vi "Turbulence_3.0.vi"() -> ()   [LabVIEW 2018]
uses:
  Quantum Composers 9000 Series.lvlib
  LightField Automation.lvclass
  Mercury iXX.lvlib
  Temperature (Read).vi
  Temperature.lvlib
  Open Temperature Device.vi
  Comms Transport Layer.ctl
  Keithley 2600 Series.lvlib
  Channel.ctl
  DAQmx Read (Counter DBL 1Chan 1Samp).vi
  Catalogue (Read).vi
  System.lvlib
  Open System.vi
panel:
  in  "File Exists":bool
  out "Log":refnum<file>
  in  "Motor free":bool
  in  "RESTART":bool
  out "time string":string
  out "Timestamp":string
  out "Log Error":errorcluster
  in  "CLOSE":bool
  in  "RECORD":bool
  in  "Turbulence":T1(tab)
  in  "New Background":bool
  out "Rate (Hz)":dbl
  out "Incident":dbl
  in  "BIN":u16(ring)=2 items=["1x1", "2x2", "4x4"]
  in  "MODE":u16(ring) items=["Normal", "DIF"]
  in  "Enable":bool
  out "Rate (Hz)":dbl
  out "Detected":dbl
  in  "Script\nEnd":u32=1 step=1
  in  "Sample Space Pump":bool
  in  "Siphon Pump":bool
  in  "Neutron Shutter":bool
  in  "Manual Script Entry (0)":string
  in  "READY":bool
  out "Power (mW)":dbl format="%_3f"
  out "Tank Pressure 2 (Torr)":string="0.0"
  in  "LIGHTFIELD":bool
  in  "SCRIPTING":bool
  in  "Top Coil":bool
  in  "# Frames":i32=1000 min=0 step=1
  in  "On CCD Acc.":i32=3 min=0 step=1
  out "Tank Pressure 1 (Torr)":string="0.0"
  out "Cell Temp (K)":dbl format="%.3f"
  in  "Data folder":path=path "C:/Data"
  out "Cryostat Temp (K)":dbl format="%.3f"
  in  "Data Interval (s)":dbl=0.5 min=0.4 max=10.0 step=0.05
  in  "RUN/STOP":bool
  in  "Bottom Coil":bool
  in  "Bottom Coil (mA)":dbl min=-1000.0 max=1000.0 step=1e-05
  in  "Top Coil (mA)":dbl min=-1000.0 max=1000.0 step=1e-05
  in  "Percent Open":i32 min=0 max=100 step=5
  in  "COOLDOWN":bool
  in  "Script\n#":i32 step=1
  in  "Kill Switch":bool
  in  "DATA":bool
  out "Scripting \nError":T2
  in  "Shutter Mode":u16(ring)=1 items=["Manual"=1, "XGate"=5]
  in  "Time (s)":i32=120 min=1 max=300 step=1
  out "Actual 3He\nTank Pressure":dbl min=0.0 max=100.0 step=5.0 format="%#.1g"
  out "Desired V2\nPressure (3He)":dbl min=0.0 max=100.0 step=5.0 format="%#.1f"
  in  "Desired Tank\nPressure (3He)":dbl min=0.0 max=100.0 step=0.01 format="%#.2f"
  in  "Log Pressure":bool
  out "4He Pressure (Torr)":string="-0.1"
  out "3He Pressure (Torr)":string="1"
  out "Temperature Error":errorcluster={"status"=TRUE, "code"=-1073807339, "source"="VISA Read in Mercury iXX.lvlib:Query (Dynamic).vit->Mercury iXX.lvlib:Query (Low Level).vi:10049->Mercury iXX.lvlib:Query.vi:3960048->Mercury iXX.lvlib:Read (Str).vi:5300004->Mercury iXX.lvlib:System.lvlib:Catalogue (Read).vi->Turbulence.vi"}
  out "File I/O Error":errorcluster
  out "4He Gauge Error":errorcluster={"status"=TRUE, "code"=-1073807343, "source"="VISA Open in Turbulence.vi"}
  out "Heater Error":errorcluster={"status"=FALSE, "code"=1073676293, "source"="VISA Read in Keithley 2600 Series.lvlib:Print Number.vi->Keithley 2600 Series.lvlib:Measure.vi->Turbulence.vi"}
  out "Pulse Generator Error":errorcluster
  out "3He Gauge Error":errorcluster={"status"=FALSE, "code"=1073676293, "source"="VISA Read in 3HeClose.vi->Turbulence.vi"}
  out "Relay Errror":errorcluster
  out "Zaber Motor Error":errorcluster
  out "LightField Error":errorcluster
  out "Shutter Error":errorcluster
  # "Camera Controls"
  # "Temperature Readout"
  # "Pressure Readout"
  # "Neutron Counts"
  # "Automation"
  # "Heater Controls"
  # "Relay Controls"
  # "Needle Valve Control"
  # "Neutron Shutter"
  # "Optical Shutter"
  # "Siphon Pump"
  # "Laser Power Meter"
  # "Sample Space\nPump"
  # "V1 = 4075 mL"
  # "V2 = 15.5 mL"
  # "V3 = 78.8 mL"
  # "Quartz\nCell"
  # "4"
  # "3psi relief"
  # "V1"
  # "4L Tank"
  # "Turbo Pump"
  # "V2"
  # "V3"
  # "3"
  # "10psi relief"
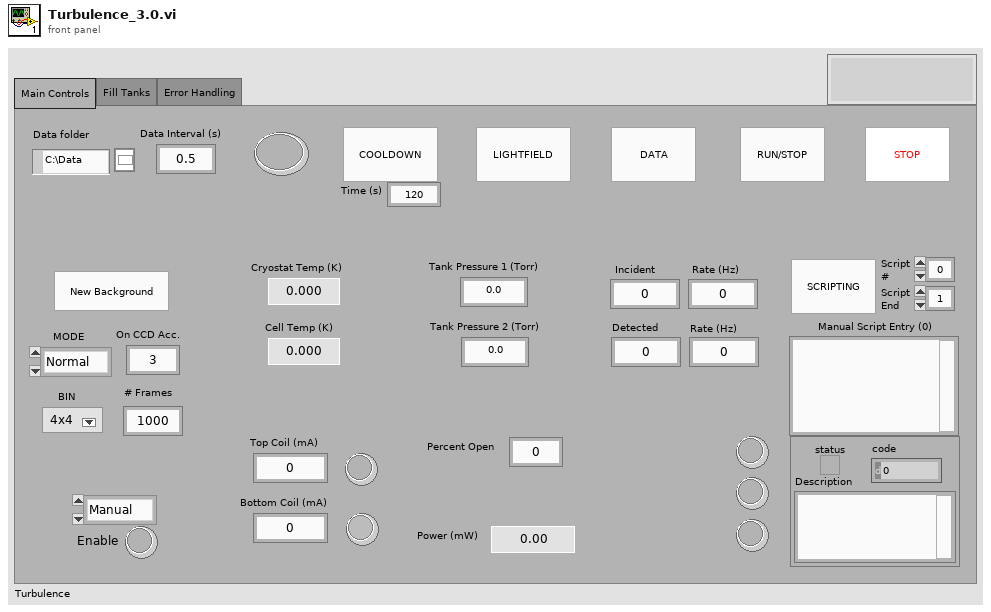
[diagram p1: front panel]
types:
  T1 = enum32{"Main Controls", "Fill Tanks", "Error Handling"}
  T2 = cluster{"status":bool, "code":i32, "Description":string}
  T3 = typedef "Mercury iXX.lvlib/Comms Transport Layer.ctl" = enum16{"Ethernet TCP/IP", "USB", "ISOBus - RS-232", "GPIB"}
  T4 = typedef "Mercury iXX.lvlib/Mercury Reference.ctl" = cluster{"Comms":refnum<visa-resource-name>, "Device ID":string[], "Comms Layer":T3, "Command":string, "Query reference":T5}
  T5 = typedef "Mercury iXX.lvlib/Query Dynamic Reference.ctl" = refnum<vi>
  T6 = enum32{"Current", "Voltage", "IV", "Resistance", "Power"}
  T7 = typedef "Keithley 2600 Series.lvlib/Channel.ctl" = enum32{"Channel A", "Channel B"}
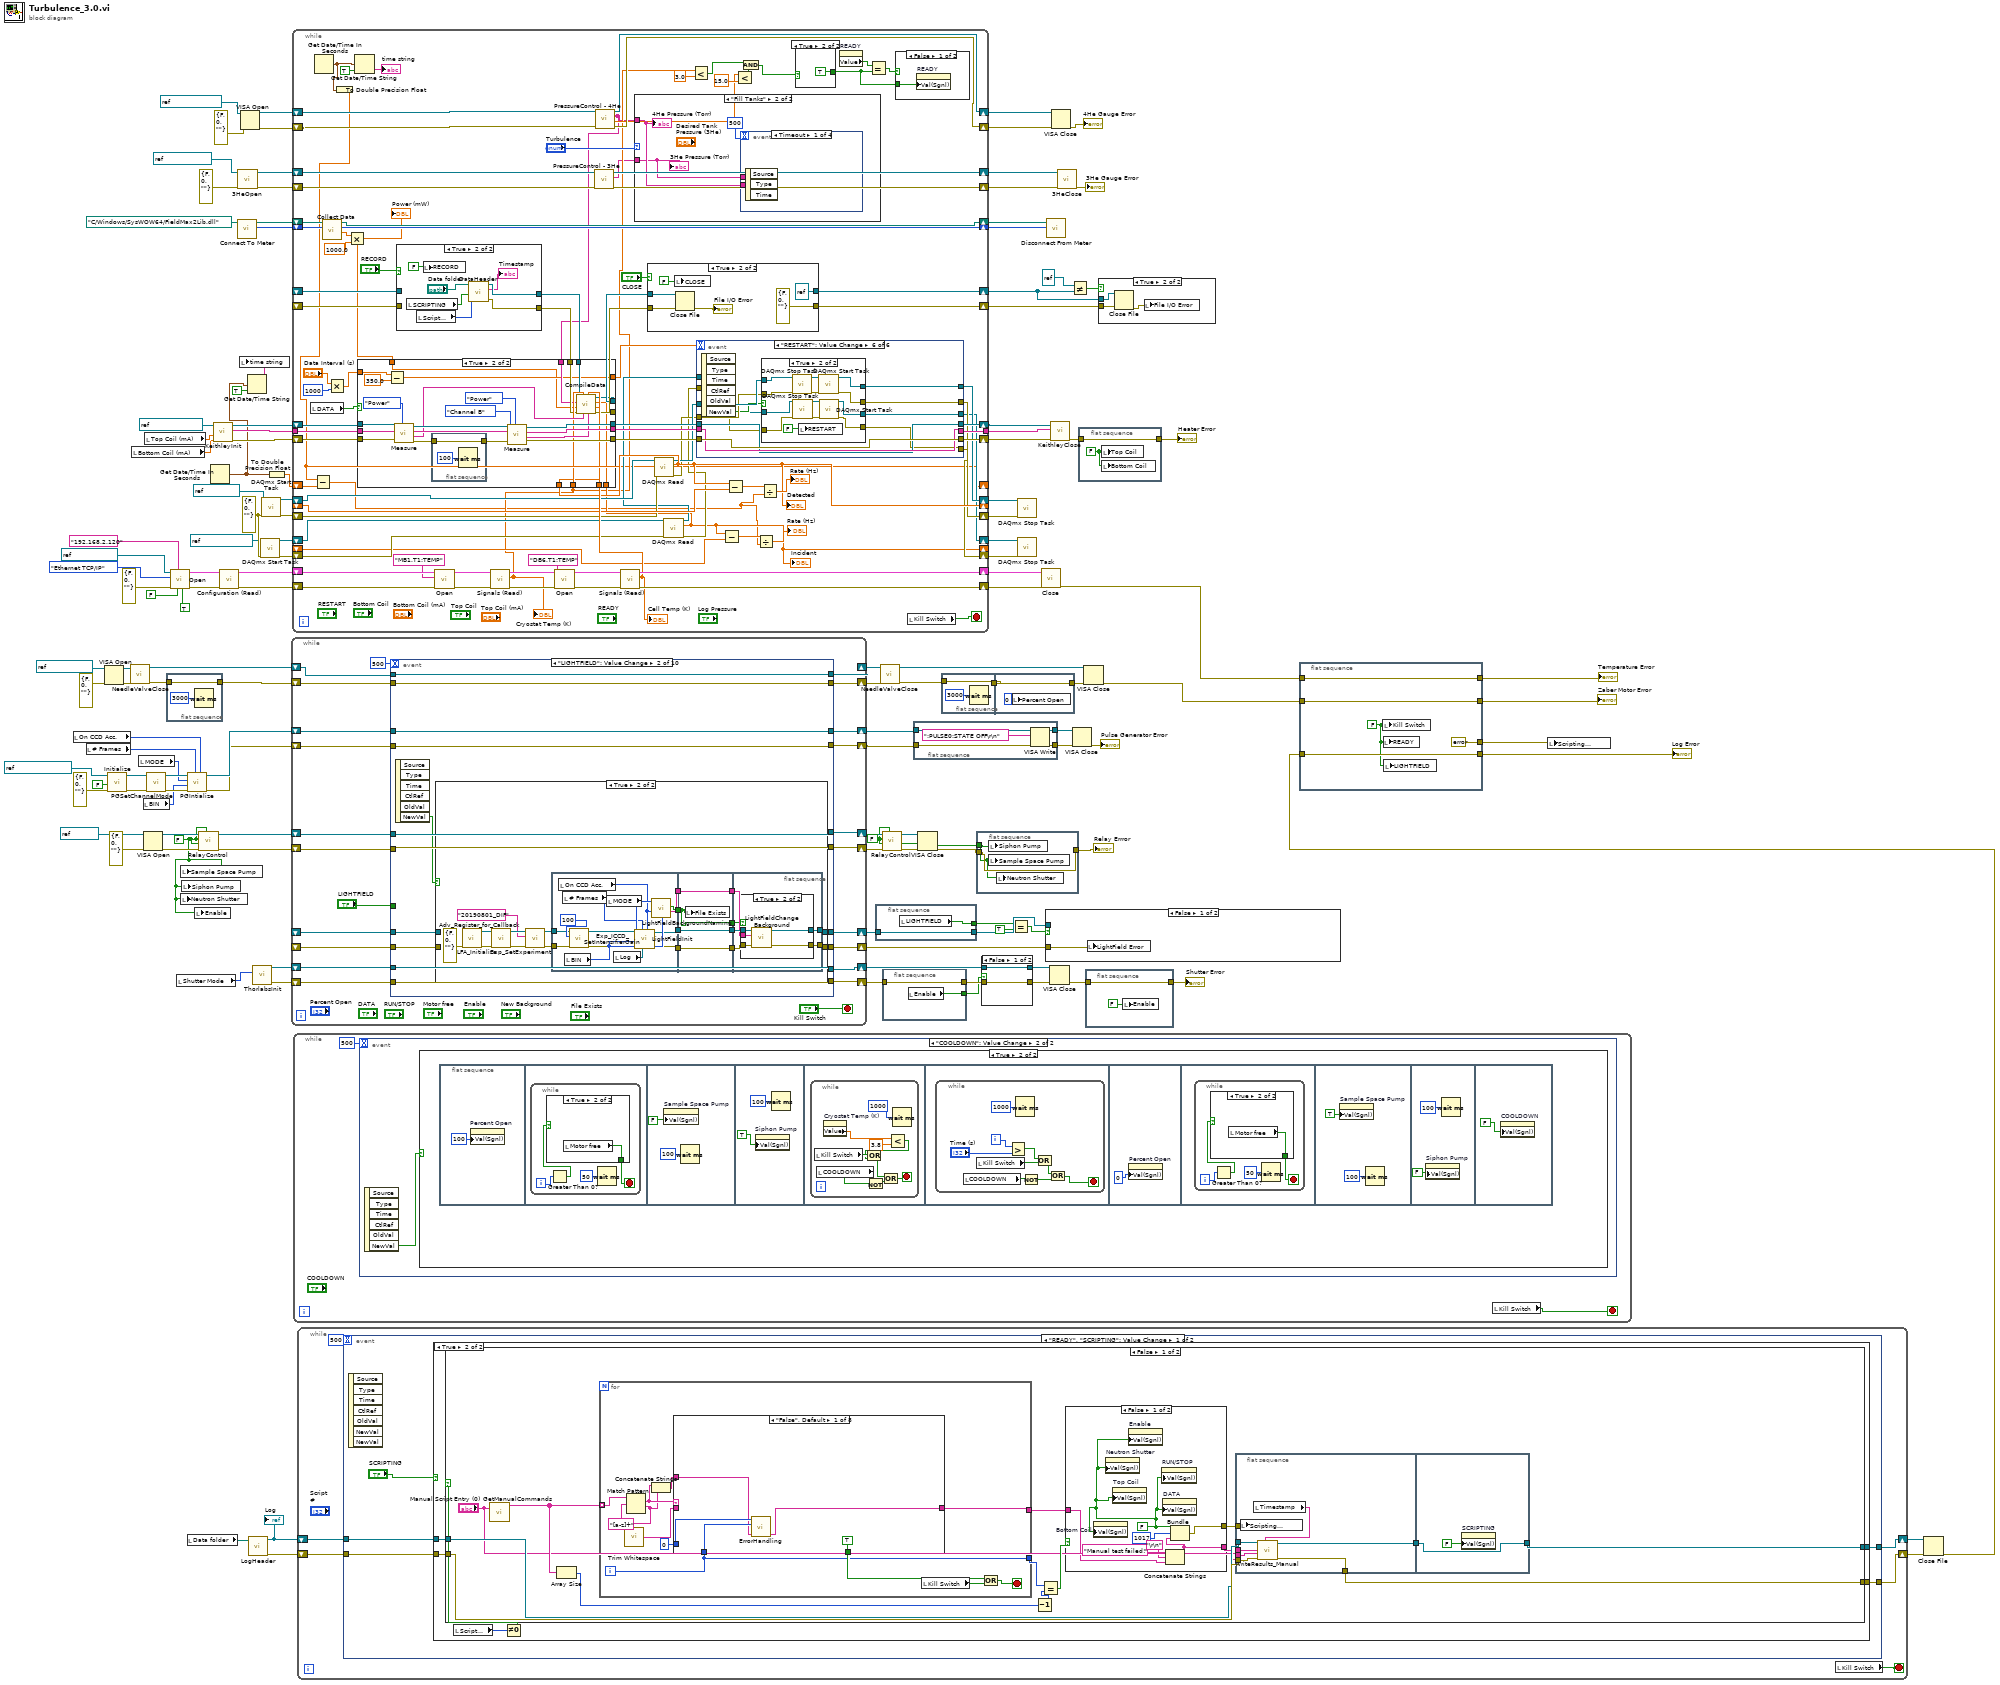
[diagram p0: block diagram]
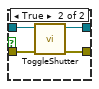
[diagram p2: hidden frame]
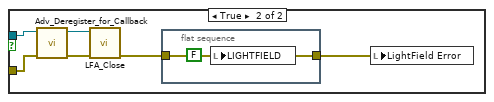
[diagram p3: hidden frame]
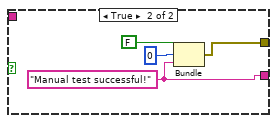
[diagram p5: hidden frame]
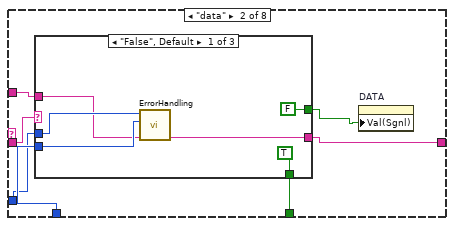
[diagram p6: hidden frame]
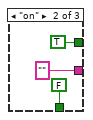
[diagram p7: hidden frame]
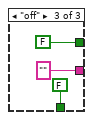
[diagram p8: hidden frame]
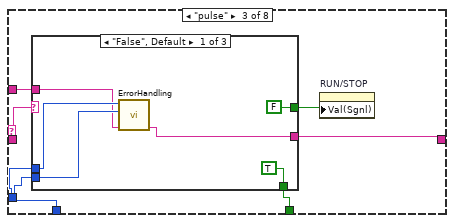
[diagram p9: hidden frame]
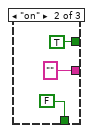
[diagram p10: hidden frame]
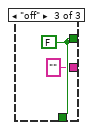
[diagram p11: hidden frame]
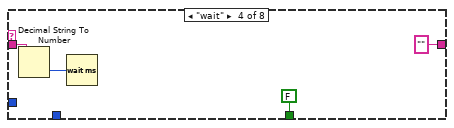
[diagram p12: hidden frame]
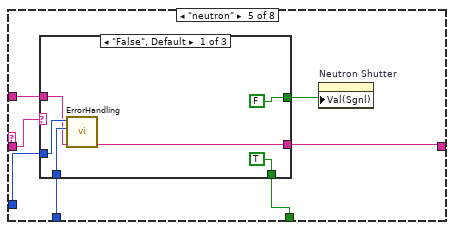
[diagram p13: hidden frame]
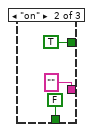
[diagram p14: hidden frame]
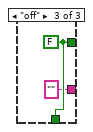
[diagram p15: hidden frame]
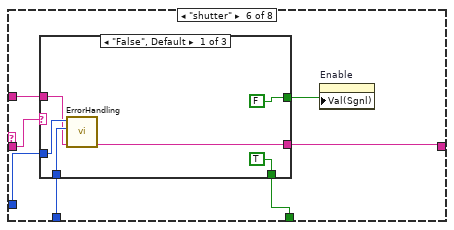
[diagram p16: hidden frame]
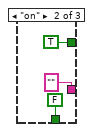
[diagram p17: hidden frame]
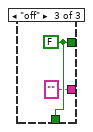
[diagram p18: hidden frame]
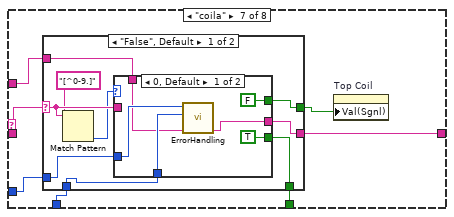
[diagram p19: hidden frame]
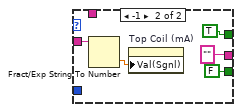
[diagram p20: hidden frame]
diagram:
  w22 = errorcluster {"status"=FALSE, "code"=0, "source"=""} ("error in")
  w60 = FALSE ("Siphon Pump")
  w44 = FALSE ("Siphon Pump")
  n1 = local read "On CCD Acc."() -> (w33:i32)
  n2 = local read "# Frames"() -> (w32:i32)
  n3 = VISA Open(error in (no error)=errorcluster {"status"=FALSE, "code"=0, "source"=""}, VISA resource name=refnum<visa-resource-name> "ZaberMotor") -> (VISA resource name=w39:refnum<visa-resource-name>, error out=w40:errorcluster)  [unwired: 3 in]
  n4 = call "Initialize.vi"("error in (no error)"=errorcluster {"status"=FALSE, "code"=0, "source"=""}, "Reset? (T: Yes)"=FALSE, "VISA resource name"=refnum<visa-resource-name> "PulseGenerator" ("Pulse generater (COM3)")) -> ("error out"=w51:errorcluster, "VISA resource name out"=w49:refnum<visa-resource-name>)  [unwired: 7 in]
  n5 = call "NeedleValveClose.vi"("error in (no error)"=w40, "VISA resource name"=w39) -> ("error out"=w41:errorcluster, "VISA resource name out"=w82:refnum<visa-resource-name>)  [unwired: 8 in]
  n6 = local read "Bottom Coil (mA)"() -> (w94:dbl)
  n7 = local read "MODE"() -> (w30:u16)
  n8 = local read "BIN"() -> (w31:u16)
  n9 = VISA Open(error in (no error)=errorcluster {"status"=FALSE, "code"=0, "source"=""} ("error in (no error) 2"), VISA resource name=refnum<visa-resource-name> "Relays" ("Pressure Gauge")) -> (VISA resource name=w107:refnum<visa-resource-name>, error out=w109:errorcluster)  [unwired: 3 in]
  n10 = local read "Top Coil (mA)"() -> (w95:dbl)
  n11 = call "PGSetChannelMode.vi"("error in"=w51, "VISA resource name"=w49) -> ("error out"=w50:errorcluster, "VISA resource name out"=w48:refnum<visa-resource-name>)  [unwired: 8 in]
  n12 = flat-sequence {
    tunnel: w41 -> [w136]
    tunnel: [w136] -> w83
    frame #0 {
      n13 = Wait (ms)(milliseconds to wait=u32 3000) -> ()  [unwired: 1 out]
    }
  }
  n14 = call-poly "Open.vi"("Clear Previous Connections (False)"=TRUE, "ID Query (True)"=FALSE, "IP Address"="192.168.2.120", "error in (no error)"=errorcluster {"status"=FALSE, "code"=0, "source"=""}, "Comms Layer"=Comms_Transport_Layer."Ethernet TCP/IP", "VISA resource name"=refnum<visa-resource-name> "MercuryiTC") -> ("error out"=w128:errorcluster, "Mercury Reference Out"=w129:T4)  [unwired: 1 in, 3 out]
  n15 = local read "Shutter Mode"() -> (w34:u16)
  n16 = local write "Sample Space Pump"(w44) -> ()
  n17 = local write "Neutron Shutter"(w44) -> ()
  n18 = local write "Siphon Pump"(w44) -> ()
  n19 = local read "Data folder"() -> (w58:path)
  n20 = call "PGIntialize.vi"("On CCD Accumulations"=w33, "Number of Frames"=w32, "error in"=w50, "BIN"=w31, "MODE"=w30, "VISA resource name"=w48) -> ("error out"=w133:errorcluster, "VISA resource name out"=w134:refnum<visa-resource-name>)  [unwired: 4 in]
  n21 = local write "Enable"(w44) -> ()
  n22 = call "RelayControl.vi"("Neutron Shutter"=w44, "Error In"=w109, "Sample Space Pump"=w44, "Siphon Pump"=w44, "Relay In"=w107) -> ("Error Out"=w108:errorcluster, "Relay Out"=w106:refnum<visa-resource-name>)  [unwired: 5 in]
  n23 = Get Date/Time In Seconds() -> (seconds since 1Jan1904=w1:timestamp)
  n24 = call "KeithleyInit.vi"("Bottom Coil (mA)"=w94, "Top Coil (mA)"=w95, "KeithleyVISA In"=refnum<visa-resource-name> "Keithley2614B" ("VISA resource name")) -> ("error out"=w98:errorcluster, "Node Out"=w99:string, "KeithleyVISA Out"=w97:refnum<visa-resource-name>)  [unwired: 6 in]
  n25 = call-poly "Configuration (Read).vi"("error in"=w128, "Mercury Reference In"=w129) -> ("error out"=w124:errorcluster, "Mercury Reference Out"=w125:T4)  [unwired: 6 in, 2 out]
  n26 = call "Connect To Meter.vi"("Location of FieldMax2Lib.dll in"=path "C:/Windows/SysWOW64/FieldMax2Lib.dll") -> ("Meter ID out"=w68:i32, "Location of FieldMax2Lib.dll out"=w67:path)  [unwired: 6 in, 1 out]
  n27 = call "3HeOpen.vi"("error in (no error)"=errorcluster {"status"=FALSE, "code"=0, "source"=""} ("error in (no error) 2"), "VISA resource name"=refnum<visa-resource-name> "3HePressure" ("Pressure Gauge")) -> ("error out"=w111:errorcluster, "VISA resource name out"=w110:refnum<visa-resource-name>)  [unwired: 8 in]
  n28 = VISA Open(error in (no error)=errorcluster {"status"=FALSE, "code"=0, "source"=""} ("error in (no error) 2"), VISA resource name=refnum<visa-resource-name> "TankPressure" ("Pressure Gauge")) -> (VISA resource name=w121:refnum<visa-resource-name>, error out=w122:errorcluster)  [unwired: 3 in]
  n29 = Get Date/Time String(seconds (now)=w1, want seconds? (F)=TRUE) -> (time string=w2:string)  [unwired: 1 in, 1 out]
  n30 = local write "time string"(w2) -> ()
  n31 = call "LogHeader.vi"("Data folder"=w58) -> ("error out"=w56:errorcluster, "refnum out"=w57:refnum<file>)  [unwired: 9 in]
  "Log" <- w57
  n32 = call "ThorlabsInit.vi"("Shutter Mode"=w34) -> ("error out"=w45:errorcluster, "VISA resource name out"=w46:refnum<visa-resource-name>)  [unwired: 9 in]
  n33 = call "DAQmx Start Task.vi"("task/channels in"=refnum<k21> "IncidentBeam", "error in"=w22) -> ("task out"=w24:refnum<k21>, "error out"=w23:errorcluster)  [unwired: 12 in]
  n34 = call "DAQmx Start Task.vi"("task/channels in"=refnum<k21> "Detector", "error in"=w22) -> ("task out"=w27:refnum<k21>, "error out"=w26:errorcluster)  [unwired: 12 in]
  n35 = To Double Precision Float(number=w1) -> (double precision float=w4:dbl)
  n36 = while {
    shift-right: [w159] -> w11
    shift-left: _ -> [w157]
    shift-right: [w160] -> w18
    shift-left: _ -> [w158]
    shift-right: [w153] -> w76
    shift-left: w134 -> [w155]
    shift-right: [w154] -> w77
    shift-left: w133 -> [w156]
    shift-right: [w149] -> w81
    shift-left: w108 -> [w152]
    shift-right: [w150] -> w79
    shift-left: w106 -> [w151]
    shift-right: [w144] -> w112
    shift-left: w83 -> [w147]
    shift-right: [w145] -> w113
    shift-left: w82 -> [w146]
    shift-right: [w141] -> w14
    shift-left: w46 -> [w138]
    shift-right: [w140] -> w7
    shift-left: w45 -> [w139]
    stop <- "Kill Switch" stop-if-true
    n37 = event shown="[1] \"LIGHTFIELD\": Value Change" {
      selector: _ -> [_ _ _ _ _ _ _ _ _ _]
      dyn-events: _ -> [_ _ _ _ _ _ _ _ _ _]
      timeout: 500 -> [_ _ _ _ _ _ _ _ _ _]
      tunnel: w156 -> [w168 w177 w253 w296 w314 w361 w424 w443 w458 w481]
      tunnel: w155 -> [w167 w176 w254 w297 w313 w362 w425 w442 w457 w480]
      tunnel: w158 -> [w169 w180 w244 w288 w316 w365 w422 w446 w462 w472]
      tunnel: w157 -> [w170 w181 w245 w289 w317 w366 w423 w447 w461 w473]
      tunnel: [w169 w182 w243 w288 w316 w353 w422 w446 w462 w472] -> w160
      tunnel: [w170 w183 w242 w289 w317 w345 w423 w447 w461 w473] -> w159
      tunnel: [w168 w177 w256 w296 w314 w351 w424 w443 w458 w478] -> w154
      tunnel: [w167 w176 w255 w297 w313 w358 w425 w442 w457 w479] -> w153
      tunnel: w152 -> [w165 w178 w250 w294 w319 w360 w431 w445 w460 w474]
      tunnel: w151 -> [w166 w179 w251 w295 w318 w359 w430 w444 w459 w475]
      tunnel: [w166 w179 w251 w295 w318 w359 w427 w444 w459 w475] -> w150
      tunnel: [w165 w178 w250 w294 w319 w360 w426 w445 w460 w474] -> w149
      tunnel: w147 -> [w164 w175 w249 w298 w302 w364 w421 w441 w456 w476]
      tunnel: w146 -> [w163 w174 w248 w299 w315 w363 w420 w440 w455 w477]
      tunnel: [w163 w174 w248 w299 w312 w363 w420 w440 w455 w477] -> w145
      tunnel: [w164 w175 w249 w298 w304 w364 w421 w441 w456 w476] -> w144
      tunnel: "LIGHTFIELD" -> [_ _ w241 w293 _ w347 _ _ _ w468]
      tunnel: w138 -> [w161 w172 w247 w291 w310 w357 w418 w439 w466 w471]
      tunnel: w139 -> [w162 w171 w246 w290 w309 w356 w417 w438 w465 w470]
      tunnel: [w161 w172 w247 w291 w310 w357 w418 w436 w463 w471] -> w141
      tunnel: [w162 w171 w246 w290 w309 w356 w417 w437 w464 w470] -> w140
      event Timeout {
        n38 = event-data() -> ()  [unwired: 1 in, 3 out]
      }
      event "LIGHTFIELD": Value Change {
        n39 = event-data() -> ("NewVal"=w173:bool)  [unwired: 1 in, 5 out]
        n40 = case shown="True" w173 {
          tunnel: [refnum<class "LightField Automation.lvclass"> refnum ("LightField Automation out") w199] -> w183
          tunnel: [errorcluster {"status"=FALSE, "code"=0, "source"=""} ("error out") w198] -> w182
          tunnel: w181 -> [w187 _]
          tunnel: w180 -> [w186 _]
          frame False {
            n41 = call "Adv_Deregister_for_Callback.vi"("error in (no error)"=w186, "LightField Automation in"=w187) -> ("error out"=w189:errorcluster, "LightField Automation out"=w190:refnum<class "LightField Automation.lvclass">)  [unwired: 8 in]
            n42 = call "LFA_Close.vi"("error in (no error)"=w189, "LightField Automation in"=w190) -> ("error out"=→"LightField Error":errorcluster)  [unwired: 8 in, 1 out]
          }
          frame True {
            n43 = call "LFA_Initialize.vi"("error in (no error)"=errorcluster {"status"=FALSE, "code"=0, "source"=""}) -> ("error out"=w208:errorcluster, "LightField Automation out"=w207:refnum<class "LightField Automation.lvclass">)  [unwired: 9 in]
            n44 = call "Adv_Register_for_Callback.vi"("error in (no error)"=w208, "LightField Automation in"=w207) -> ("error out"=w206:errorcluster, "LightField Automation out"=w205:refnum<class "LightField Automation.lvclass">)  [unwired: 8 in]
            n45 = call "Exp_SetExperiment.vi"("error in (no error)"=w206, "ExperimentName"="20190801_DIF", "LightField Automation in"=w205) -> ("error out"=w192:errorcluster, "LightField Automation out"=w191:refnum<class "LightField Automation.lvclass">)  [unwired: 7 in]
            n46 = flat-sequence {
              tunnel: [w211] -> w196
              tunnel: [w210] -> w195
              tunnel: [w209] -> w194
              tunnel: [w212] -> w193
              tunnel: w192 -> [w215]
              tunnel: w191 -> [w213]
              tunnel: [w226] -> w202
              tunnel: [w225] -> w201
              tunnel: [w224] -> w200
              tunnel: [w223] -> w197
              tunnel: w196 -> [w223]
              tunnel: w195 -> [w226]
              tunnel: w194 -> [w225]
              tunnel: w193 -> [w224]
              tunnel: w202 -> [w231]
              tunnel: w201 -> [w232]
              tunnel: w200 -> [w230]
              tunnel: [w229] -> w199
              tunnel: [w228] -> w198
              tunnel: w197 -> [w227]
              frame #0 {
                n47 = local read "On CCD Acc."() -> (w221:i32)
                n48 = local read "# Frames"() -> (w219:i32)
                n49 = local read "BIN"() -> (w220:u16)
                n50 = call "Exp_ICCD_SetIntensifierGain.vi"("error in (no error)"=w215, "Intensifier Gain"=100, "LightField Automation in"=w213) -> ("error out"=w217:errorcluster, "LightField Automation out"=w216:refnum<class "LightField Automation.lvclass">)  [unwired: 7 in]
                n51 = local read "MODE"() -> (w222:u16)
                n52 = local read "Log"() -> (w218:refnum<file>)
                n53 = call "LightFieldInit.vi"("On CCD Accumulations"=w221, "File Path"=w218, "Number of Frames"=w219, "error in"=w217, "BIN"=w220, "MODE"=w222, "LightField Automation in"=w216) -> ("error out"=w210:errorcluster, "LightField Automation out"=w209:refnum<class "LightField Automation.lvclass">)  [unwired: 3 in]
                n54 = call "LightFieldBackgroundNaming.vi"("On CCD Acc."=w221, "BIN"=w220, "MODE"=w222) -> ("FilePath"=w212:string, "Exists"=w211:bool)  [unwired: 6 in, 1 out]
              }
              frame #1 {
                n55 = local write "File Exists"(w223) -> ()
              }
              frame #2 {
                n56 = case shown="True" w227 {
                  tunnel: w232 -> [w235 w240]
                  tunnel: w231 -> [w234 w239]
                  tunnel: w230 -> [_ w238]
                  tunnel: [w235 w237] -> w229
                  tunnel: [w234 w236] -> w228
                  frame False {
                    n57 = property on="New Background" class="Bool (strict)"("Val(Sgnl)"=TRUE ("Value (Signaling)")) -> ()  [unwired: 2 in, 2 out]
                  }
                  frame True {
                    n58 = call "LightFieldChangeBackground.vi"("error in"=w239, "FilePath"=w238, "LightField Automation in"=w240) -> ("error out"=w236:errorcluster, "LightField Automation out"=w237:refnum<class "LightField Automation.lvclass">)  [unwired: 7 in]
                  }
                }
              }
            }
          }
        }
      }
      event "RUN/STOP": Value Change {
        n59 = event-data() -> ("NewVal"=w252:bool)  [unwired: 1 in, 5 out]
        n60 = case shown="False" w252 {
          tunnel: [w260 w273] -> w256
          tunnel: [w261 w272] -> w255
          tunnel: w254 -> [w262 w271]
          tunnel: w253 -> [w263 w270]
          tunnel: w245 -> [w258 w268]
          tunnel: w244 -> [w257 w267]
          tunnel: [w257 w266] -> w243
          tunnel: [w258 w265] -> w242
          tunnel: w241 -> [_ w264]
          frame False {
            n61 = VISA Write(VISA resource name=w262, write buffer=":PULSE0:STATE OFF\r\n" ("format string"), error in (no error)=w263) -> (VISA resource name out=w261:refnum<visa-resource-name>, error out=w260:errorcluster)  [unwired: 1 out]
          }
          frame True {
            n62 = case shown="True" w264 {
              tunnel: w267 -> [w274 w283]
              tunnel: w268 -> [w275 w281]
              tunnel: [w275 w285] -> w265
              tunnel: [w274 w284] -> w266
              frame False {
              }
              frame True {
                n63 = local read "MODE"() -> (w278:u16)
                n64 = local read "SCRIPTING"() -> (w276:bool)
                n65 = local read "BIN"() -> (w279:u16)
                n66 = case shown="True" w276 {
                  tunnel: [-1 ("Script\n#") w287] -> w277
                  frame False {
                  }
                  frame True {
                    n67 = local read "Script\n#"() -> (w287:i32)
                  }
                }
                n68 = call "LightFieldFileNaming.vi"("Script#"=w277, "error in"=w283, "BIN"=w279, "MODE"=w278, "LightField Automation in"=w281) -> ("error out"=w282:errorcluster, "LightField Automation out"=w280:refnum<class "LightField Automation.lvclass">)  [unwired: 5 in]
                n69 = call "LFA_Acquire.vi"("error in (no error)"=w282, "LightField Automation in"=w280) -> ("error out"=w284:errorcluster, "LightField Automation out"=w285:refnum<class "LightField Automation.lvclass">)  [unwired: 8 in]
              }
            }
            n70 = VISA Write(VISA resource name=w271, write buffer=":PULSE0:STATE ON\r\n" ("format string"), error in (no error)=w270) -> (VISA resource name out=w272:refnum<visa-resource-name>, error out=w273:errorcluster)  [unwired: 1 out]
          }
        }
      }
      event "DATA": Value Change {
        n71 = event-data() -> ("NewVal"=w292:bool)  [unwired: 1 in, 5 out]
        n72 = case shown="True" w292 {
          tunnel: w293 -> [_ _]
          frame False {
            n73 = local write "CLOSE"(TRUE ("CLOSE")) -> ()
          }
          frame True {
            n74 = local write "RECORD"(TRUE ("RECORD")) -> ()
          }
        }
      }
      event "Percent Open": Value Change {
        n75 = event-data() -> ("OldVal"=w311:i32, "NewVal"=w320:i32)  [unwired: 1 in, 4 out]
        n76 = flat-sequence {
          tunnel: w302 -> [w322]
          tunnel: [w322] -> w303
          frame #0 {
            n77 = property on="Motor free" class="Bool (strict)"("Val(Sgnl)"=FALSE ("Value (Signaling)")) -> ()  [unwired: 2 in, 2 out]
          }
        }
        n78 = Subtract(x=w320, y=w311) -> (x-y=w306:i32)
        n79 = Greater Than 0?(x=w306) -> (x > 0?=w307:bool)
        n80 = Equal To 0?(x=w320) -> (x = 0?=w308:bool)
        n81 = case shown="False" w308 {
          tunnel: w315 -> [w328 w344]
          tunnel: w303 -> [w329 w343]
          tunnel: [w327 w342] -> w312
          tunnel: [w326 w341] -> w305
          tunnel: w307 -> [w330 _]
          tunnel: w306 -> [w325 _]
          frame False {
            n82 = case shown="True" w330 {
              tunnel: w329 -> [w334 w340]
              tunnel: w328 -> [w335 w339]
              tunnel: [w333 w338] -> w327
              tunnel: [w332 w337] -> w326
              tunnel: w325 -> [w331 w336]
              frame False {
                n83 = call "NeedleValveClose - Encoder.vi"("error in (no error)"=w334, "Percent Difference"=w331, "VISA resource name"=w335) -> ("error out"=w332:errorcluster, "VISA resource name out"=w333:refnum<visa-resource-name>)  [unwired: 7 in]
              }
              frame True {
                n84 = call "NeedleValveOpen - Encoder.vi"("error in (no error)"=w340, "Percent Difference"=w336, "VISA resource name"=w339) -> ("error out"=w337:errorcluster, "VISA resource name out"=w338:refnum<visa-resource-name>)  [unwired: 7 in]
              }
            }
          }
          frame True {
            n85 = call "NeedleValveClose.vi"("error in (no error)"=w343, "VISA resource name"=w344) -> ("error out"=w341:errorcluster, "VISA resource name out"=w342:refnum<visa-resource-name>)  [unwired: 8 in]
          }
        }
        n86 = flat-sequence {
          tunnel: w305 -> [w324]
          tunnel: [w324] -> w304
          frame #0 {
            n87 = property on="Motor free" class="Bool (strict)"("Val(Sgnl)"=TRUE ("Value (Signaling)")) -> ()  [unwired: 2 in, 2 out]
          }
        }
      }
      event "On CCD Acc.", "# Frames", "MODE", "BIN": Value Change {
        n88 = event-data() -> ()  [unwired: 1 in, 4 out]
        n89 = case shown="True" w347 {
          tunnel: w366 -> [w405 w413]
          tunnel: w365 -> [w406 w414]
          tunnel: [w405 w412] -> w346
          tunnel: [w406 w411] -> w354
          tunnel: "On CCD Acc." -> [_ w409]
          tunnel: "# Frames" -> [_ w410]
          tunnel: "BIN" -> [_ w408]
          tunnel: "MODE" -> [_ w407]
          frame False {
          }
          frame True {
            n90 = call "LightFieldParams.vi"("On CCD Accumulations"=w409, "Number of Frames"=w410, "error in"=w414, "BIN"=w408, "MODE"=w407, "LightField Automation in"=w413) -> ("error out"=w411:errorcluster, "LightField Automation out"=w412:refnum<class "LightField Automation.lvclass">)  [unwired: 4 in]
          }
        }
        n91 = call "PGIntialize.vi"("On CCD Accumulations"="On CCD Acc.", "Number of Frames"="# Frames", "error in"=w361, "BIN"="BIN", "MODE"="MODE", "VISA resource name"=w362) -> ("error out"=w352:errorcluster, "VISA resource name out"=w358:refnum<visa-resource-name>)  [unwired: 4 in]
        n92 = case shown="True" w347 {
          tunnel: w354 -> [w369 w378]
          tunnel: [w369 w377] -> w353
          tunnel: w352 -> [w368 w376]
          tunnel: [w368 w375] -> w351
          tunnel: "On CCD Acc." -> [_ w374]
          tunnel: "BIN" -> [_ w373]
          tunnel: "MODE" -> [_ w372]
          tunnel: w346 -> [w367 w371]
          tunnel: [w367 w370] -> w345
          frame False {
          }
          frame True {
            n93 = flat-sequence {
              tunnel: w378 -> [w381]
              tunnel: [w380] -> w377
              tunnel: w376 -> [w389]
              tunnel: [w389] -> w375
              tunnel: w374 -> [w388]
              tunnel: w373 -> [w387]
              tunnel: w372 -> [w386]
              tunnel: w371 -> [w382]
              tunnel: [w379] -> w370
              frame #0 {
                n94 = call "LightFieldBackgroundNaming.vi"("On CCD Acc."=w388, "BIN"=w387, "MODE"=w386) -> ("FilePath"=w383:string, "Exists"=w385:bool)  [unwired: 6 in, 1 out]
                n95 = flat-sequence {
                  tunnel: w385 -> [w390]
                  tunnel: [w390] -> w384
                  tunnel: w384 -> [w396]
                  tunnel: w383 -> [w395]
                  tunnel: w382 -> [w394]
                  tunnel: w381 -> [w393]
                  tunnel: [w392] -> w380
                  tunnel: [w391] -> w379
                  frame #0 {
                    n96 = local write "File Exists"(w390) -> ()
                  }
                  frame #1 {
                    n97 = case shown="False" w396 {
                      tunnel: w395 -> [_ w404]
                      tunnel: w394 -> [w398 w403]
                      tunnel: w393 -> [w397 w402]
                      tunnel: [w397 w401] -> w392
                      tunnel: [w398 w400] -> w391
                      frame False {
                        n98 = property on="New Background" class="Bool (strict)"("Val(Sgnl)"=TRUE ("Value (Signaling)")) -> ()  [unwired: 2 in, 2 out]
                      }
                      frame True {
                        n99 = call "LightFieldChangeBackground.vi"("error in"=w402, "FilePath"=w404, "LightField Automation in"=w403) -> ("error out"=w401:errorcluster, "LightField Automation out"=w400:refnum<class "LightField Automation.lvclass">)  [unwired: 7 in]
                      }
                    }
                  }
                }
              }
            }
          }
        }
      }
      event "Siphon Pump", "Sample Space Pump", "Neutron Shutter": Value Change {
        n100 = event-data() -> ("CtlRef"=w416:refnum<vi>)  [unwired: 1 in, 5 out]
        n101 = property class="Bool (strict)"(reference=w416) -> ("Label.Text"=w415:string)  [unwired: 1 in, 2 out]
        n102 = call "RelayControl.vi"("Neutron Shutter"="Neutron Shutter", "Error In"=w431, "Sample Space Pump"="Sample Space Pump", "Siphon Pump"="Siphon Pump", "Relay In"=w430) -> ("Error Out"=w426:errorcluster, "Relay Out"=w427:refnum<visa-resource-name>)  [unwired: 5 in]
        n103 = case shown="\"Neutron Shutter\"" w415 {
          frame "0", Default {
          }
          frame "Neutron Shutter" {
            n104 = property on="RESTART" class="Bool (strict)"("Val(Sgnl)"=TRUE ("RESTART")) -> ()  [unwired: 2 in, 2 out]
          }
        }
      }
      event "Enable": Value Change {
        n105 = event-data() -> ("OldVal"=w434:bool, "NewVal"=w435:bool)  [unwired: 1 in, 4 out]
        n106 = Not Equal?(x=w434, y=w435) -> (x != y?=w433:bool)
        n107 = case shown="True" w433 {
          tunnel: w439 -> [w449 w453]
          tunnel: w438 -> [w448 w452]
          tunnel: [w448 w451] -> w437
          tunnel: [w449 w450] -> w436
          frame False {
          }
          frame True {
            n108 = call "ToggleShutter.vi"("error in"=w452, "VISA resource name"=w453) -> ("error out"=w451:errorcluster, "VISA resource name out"=w450:refnum<visa-resource-name>)  [unwired: 8 in]
          }
        }
      }
      event "Shutter Mode": Value Change {
        n109 = event-data() -> ()  [unwired: 1 in, 6 out]
        n110 = call "ThorlabsMode.vi"("error in"=w465, "Mode"="Shutter Mode", "VISA resource name"=w466) -> ("error out"=w464:errorcluster, "VISA resource name out"=w463:refnum<visa-resource-name>)  [unwired: 7 in]
      }
      event "New Background": Value Change {
        n111 = event-data() -> ("NewVal"=w469:bool)  [unwired: 1 in]
        n112 = And(x=w469, y=w468) -> (x .and. y?=w467:bool)
        n113 = case shown="True" w467 {
          tunnel: w481 -> [w482 w493]
          tunnel: w480 -> [w483 w494]
          tunnel: [w483 w491] -> w479
          tunnel: [w482 w485] -> w478
          frame False {
          }
          frame True {
            n114 = local read "On CCD Acc."() -> (w492:i32)
            n115 = local read "MODE"() -> (w488:u16)
            n116 = local read "File Exists"() -> (w484:bool)
            n117 = local read "BIN"() -> (w487:u16)
            n118 = call "LightFieldAcquireBackground.vi"("File Exists"=w484, "On CCD Acc."=w492, "error in"=w493, "BIN"=w487, "MODE"=w488, "VISA resource name"=w494) -> ("error out"=w490:errorcluster, "VISA resource name out"=w489:refnum<visa-resource-name>)  [unwired: 4 in]
            n119 = call "PGResetCameraWait.vi"("error in"=w490, "BIN"=w487, "MODE"=w488, "VISA resource name"=w489) -> ("error out"=w486:errorcluster, "VISA resource name out"=w491:refnum<visa-resource-name>)  [unwired: 6 in]
            n120 = flat-sequence {
              tunnel: w486 -> [w496]
              tunnel: [w496] -> w485
              frame #0 {
                n121 = local write "New Background"(FALSE ("New Background")) -> ()
                n122 = local write "File Exists"(TRUE ("File Exists")) -> ()
              }
            }
          }
        }
      }
    }
  }
  n123 = while {
    shift-right: [w588] -> w126
    shift-left: w125 -> [w587]
    shift-right: [w589] -> w127
    shift-left: w124 -> [w586]
    shift-right: [w583] -> w117
    shift-left: w122 -> [w585]
    shift-right: [w582] -> w116
    shift-left: w121 -> [w584]
    shift-right: [w581] -> w62
    shift-left: _ -> [w579]
    shift-right: [w580] -> w61
    shift-left: _ -> [w578]
    shift-right: [w575] -> w86
    shift-left: w97 -> [w577]
    shift-right: [w574] -> w88
    shift-left: w98 -> [w573]
    shift-right: [w571] -> w101
    shift-left: w111 -> [w572]
    shift-right: [w569] -> w102
    shift-left: w110 -> [w570]
    tunnel: w99 -> [w576]
    tunnel: [w545] -> w87
    shift-right: [w542] -> w66
    shift-left: w68 -> [w544]
    shift-right: [w541] -> w65
    shift-left: w67 -> [w543]
    shift-right: [w530] -> _
    shift-left: _ -> [w534]
    shift-right: [w529] -> w28
    shift-left: w26 -> [w526]
    shift-right: [w528] -> w29
    shift-left: w27 -> [w527]
    shift-right: [w520] -> w20
    shift-left: w24 -> [w523]
    shift-right: [w521] -> w19
    shift-left: w23 -> [w522]
    shift-right: [w514] -> _
    shift-left: _ -> [w516]
    shift-right: [w498] -> _
    shift-left: w4 -> [w500]
    stop <- w535 stop-if-true
    n124 = local read "DATA"() -> (w540:bool)
    n125 = Get Date/Time In Seconds() -> (seconds since 1Jan1904=w502:timestamp)
    n126 = call "Collect Data.vi"("Location of FieldMax2Lib.dll in"=w543, "Meter ID in"=w544) -> ("Location of FieldMax2Lib.dll out"=w541:path, "Meter ID out"=w542:i32, "Measurement"=w538:sgl)  [unwired: 5 in, 1 out]
    n127 = Multiply(x="Data Interval (s)", y=u32 1000 ("millisecond multiple")) -> (x*y=w546:dbl)
    n128 = To Double Precision Float(number=w502) -> (double precision float=w498:dbl)
    n129 = Subtract(x=w498, y=w500) -> (x-y=w499:dbl)
    n130 = Multiply(x=w538, y=1000.0) -> (x*y=w537:dbl)
    "Power (mW)" <- w537
    n131 = Get Date/Time String(seconds (now)=w502, want seconds? (F)=TRUE) -> (time string=→"time string":string)  [unwired: 1 in, 1 out]
    n132 = case shown="True" "RECORD" {
      tunnel: w579 -> [w637 _]
      tunnel: w578 -> [w638 _]
      tunnel: [w638 w643] -> w549
      tunnel: [w637 w642] -> w550
      frame False {
      }
      frame True {
        n133 = local read "SCRIPTING"() -> (w641:bool)
        n134 = local read "Script\n#"() -> (w640:i32)
        n135 = local write "RECORD"(FALSE ("RECORD")) -> ()
        n136 = call "DataHeader.vi"("Script #"=w640, "Scripting"=w641, 11:"Data folder") -> ("error out"=w642:errorcluster, "Timestamp"=→"Timestamp":string, "refnum out"=w643:refnum<file>)  [unwired: 6 in]
      }
    }
    n137 = call-poly "Open.vi"("error in (no error)"=w586, "Device Identifier"="MB1.T1:TEMP", "Mercury Reference In"=w587) -> ("error out"=w562:errorcluster, "Mercury Reference Out"=w561:T4)  [unwired: 7 in]
    n138 = call-poly "Signals (Read).vi"("error in"=w562, "Mercury Reference In"=w561) -> ("error out"=w559:errorcluster, "Temperature"=w510:dbl, "Mercury Reference Out"=w560:T4)  [unwired: 5 in, 2 out]
    "Cryostat Temp (K)" <- w510
    n139 = call-poly "Open.vi"("error in (no error)"=w559, "Device Identifier"="DB6.T1:TEMP", "Mercury Reference In"=w560) -> ("error out"=w557:errorcluster, "Mercury Reference Out"=w558:T4)  [unwired: 7 in]
    n140 = call "PressureControl - 3He.vi"("error in (no error)"=w572, "VISA resource name"=w570) -> ("error out"=w571:errorcluster, "3HePressure (Torr)"=w504:string, "VISA resource name out"=w569:refnum<visa-resource-name>)  [unwired: 7 in]
    n141 = call "PressureControl - 4He.vi"("error in (no error)"=w585, "VISA resource name"=w584) -> ("error out"=w583:errorcluster, "Pressure"=w552:dbl, "Pressure (Torr)"=w505:string, "VISA resource name out"=w582:refnum<visa-resource-name>)  [unwired: 6 in]
    n142 = call-poly "Signals (Read).vi"("error in"=w557, "Mercury Reference In"=w558) -> ("error out"=w589:errorcluster, "Temperature"=w551:dbl, "Mercury Reference Out"=w588:T4)  [unwired: 5 in, 2 out]
    "Cell Temp (K)" <- w551
    n143 = case shown="\"Fill Tanks\"" "Turbulence" {
      tunnel: w505 -> [w646 w649]
      tunnel: w504 -> [w647 w648]
      frame "Main Controls", Default {
        "Tank Pressure 2 (Torr)" <- w647
        "Tank Pressure 1 (Torr)" <- w646
      }
      frame "Fill Tanks" {
        n144 = event shown="[0] Timeout" {
          selector: _ -> [_ _ _ _]
          dyn-events: _ -> [_ _ _ _]
          timeout: 500 ("Numeric") -> [_ _ _ _]
          tunnel: w648 -> [_ _ _ w655]
          tunnel: w649 -> [_ _ _ w657]
          event Timeout {
            n145 = event-data() -> ()  [unwired: 1 in, 3 out]
          }
          event "Desired Tank\nPressure (3He)": Value Change {
            n146 = event-data() -> ("NewVal"=w651:dbl)  [unwired: 1 in]
            n147 = call "3HePressureCalculator.vi"("Desired Tank\nPressure (3He)"=w651) -> ("V2 Pressure (3He)"=→"Desired V2\nPressure (3He)":dbl)  [unwired: 10 in]
          }
          event "3He Pressure (Torr)": Value Change {
            n148 = event-data() -> ("NewVal"=w653:string)  [unwired: 1 in]
            n149 = call "3HeActualPressure.vi"("3He Pressure (Torr)"=w653) -> ("Actual 3He\nTank Pressure"=→"Actual 3He\nTank Pressure":dbl)  [unwired: 10 in]
          }
          event "Log Pressure": Value Change {
            n150 = event-data() -> ("NewVal"=w656:bool)  [unwired: 1 in, 1 out]
            n151 = call "SaveTankData.vi"("Log Pressure"=w656, "4He Pressure (Torr)"=w657, "3He Pressure (Torr)"=w655) -> ()  [unwired: 8 in]
          }
        }
        "3He Pressure (Torr)" <- w648
        "4He Pressure (Torr)" <- w649
      }
    }
    n152 = call-poly "DAQmx Read.vi"("task/channels in"=w527, "error in"=w526) -> ("task out"=w525:refnum<k21>, "data"=w530:dbl, "error out"=w524:errorcluster)  [unwired: 11 in]
    "Detected" <- w530
    n153 = call-poly "DAQmx Read.vi"("task/channels in"=w523, "error in"=w522) -> ("task out"=w519:refnum<k21>, "data"=w514:dbl, "error out"=w518:errorcluster)  [unwired: 11 in]
    "Incident" <- w514
    n154 = case shown="True" w540 {
      tunnel: w573 -> [w596 w626]
      tunnel: w577 -> [w598 w625]
      tunnel: w576 -> [w597 w624]
      tunnel: [w597 w620] -> w556
      tunnel: [w596 w619] -> w555
      tunnel: [w598 w618] -> w554
      tunnel: w551 -> [_ w612]
      tunnel: w510 -> [_ w610]
      tunnel: w550 -> [w594 w609]
      tunnel: w505 -> [_ w608]
      tunnel: w549 -> [w595 w607]
      tunnel: [w594 w606] -> w548
      tunnel: [w595 w605] -> w547
      tunnel: w546 -> [w593 w603]
      tunnel: [w593 w602] -> w536
      tunnel: w537 -> [_ w601]
      tunnel: w530 -> [_ w600]
      tunnel: w514 -> [_ w599]
      frame False {
      }
      frame True {
        n155 = Subtract(x=w603, y=350.0) -> (x-y=w602:dbl)
        n156 = call "Measure.vi"("Function (Current)"=T6."Power", "error in (no error)"=w626, "Node In"=w624, "VISA resource name"=w625) -> ("error out"=w617:errorcluster, "Output"=w611:string, "Node Out"=w621:string, "VISA resource name out"=w622:refnum<visa-resource-name>)  [unwired: 3 in, 1 out]
        n157 = flat-sequence {
          tunnel: w617 -> [w627]
          tunnel: [w627] -> w616
          frame #0 {
            n158 = Wait (ms)(milliseconds to wait=u32 100) -> ()  [unwired: 1 out]
          }
        }
        n159 = call "Measure.vi"("Function (Current)"=T6."Power", "error in (no error)"=w616, "Channel (Channel A)"=Channel."Channel B", "Node In"=w621, "VISA resource name"=w622) -> ("error out"=w619:errorcluster, "Output"=w613:string, "Node Out"=w620:string, "VISA resource name out"=w618:refnum<visa-resource-name>)  [unwired: 2 in, 1 out]
        n160 = call "CompileData.vi"("Detected"=w600, "Incident"=w599, "Ch. B (W)"=w613, "Cell Temp (K)"=w612, "Ch. A (W)"=w611, "Cryostat Temp (K)"=w610, "error in"=w609, "Laser Power (W)"=w601, "Tank Pressure (Torr)"=w608, "refnum in"=w607) -> ("error out"=w606:errorcluster, "refnum out"=w605:refnum<file>)
      }
    }
    n161 = case shown="True" "CLOSE" {
      tunnel: w548 -> [w629 w635]
      tunnel: w547 -> [w630 w634]
      tunnel: [w630 refnum<file> refnum ("refnum out")] -> w580
      tunnel: [w629 errorcluster {"status"=FALSE, "code"=0, "source"=""} ("error out")] -> w581
      frame False {
      }
      frame True {
        n162 = local write "CLOSE"(FALSE ("CLOSE")) -> ()
        n163 = Close File(refnum=w634, error in=w635) -> (error out=→"File I/O Error":errorcluster)  [unwired: 1 out]
      }
    }
    n164 = Less?(x=w510, y=3.0) -> (x < y?=w507:bool)
    n165 = event shown="[5] \"RESTART\": Value Change" {
      selector: _ -> [_ _ _ _ _ _]
      dyn-events: _ -> [_ _ _ _ _ _]
      timeout: w536 -> [_ _ _ _ _ _]
      tunnel: w556 -> [w662 w676 w688 w700 w712 w725]
      tunnel: w555 -> [w663 w677 w690 w702 w714 w726]
      tunnel: w554 -> [w664 w675 w687 w699 w711 w724]
      tunnel: [w664 w674 w689 w701 w713 w724] -> w575
      tunnel: [w663 w670 w683 w697 w708 w726] -> w574
      tunnel: [w662 w669 w682 w696 w707 w725] -> w545
      tunnel: [w661 w668 w681 w695 w706 w723] -> w529
      tunnel: [w660 w667 w680 w694 w705 w722] -> w528
      tunnel: w525 -> [w660 w667 w680 w694 w705 w721]
      tunnel: w524 -> [w661 w668 w681 w695 w706 w720]
      tunnel: [w659 w666 w679 w693 w704 w718] -> w520
      tunnel: [w658 w665 w678 w692 w703 w717] -> w521
      tunnel: w519 -> [w659 w666 w679 w693 w704 w716]
      tunnel: w518 -> [w658 w665 w678 w692 w703 w715]
      event Timeout {
        n166 = event-data() -> ()  [unwired: 1 in, 3 out]
      }
      event "Top Coil (mA)": Value Change {
        n167 = event-data() -> ("NewVal"=w672:dbl)  [unwired: 1 in, 5 out]
        n168 = Divide(x=w672, y=1000.0) -> (x/y=w671:dbl)
        n169 = call "Source Level.vi"("Level (0.000)"=w671, "error in (no error)"=w677, "Node In"=w676, "VISA resource name"=w675) -> ("error out"=w670:errorcluster, "Node Out"=w669:string, "VISA resource name out"=w674:refnum<visa-resource-name>)  [unwired: 4 in, 1 out]
      }
      event "Bottom Coil (mA)": Value Change {
        n170 = event-data() -> ("NewVal"=w685:dbl)  [unwired: 1 in, 5 out]
        n171 = Divide(x=w685, y=1000.0) -> (x/y=w684:dbl)
        n172 = call "Source Level.vi"("Level (0.000)"=w684, "error in (no error)"=w690, "Channel (Channel A)"=Channel."Channel B", "Node In"=w688, "VISA resource name"=w687) -> ("error out"=w683:errorcluster, "Node Out"=w682:string, "VISA resource name out"=w689:refnum<visa-resource-name>)  [unwired: 3 in, 1 out]
      }
      event "Top Coil": Value Change {
        n173 = event-data() -> ("NewVal"=w698:bool)  [unwired: 1 in, 5 out]
        n174 = call "Source Output Enable.vi"("Output (Off)"=w698, "error in (no error)"=w702, "Node In"=w700, "VISA resource name"=w699) -> ("error out"=w697:errorcluster, "Node Out"=w696:string, "VISA resource name out"=w701:refnum<visa-resource-name>)  [unwired: 4 in, 1 out]
      }
      event "Bottom Coil": Value Change {
        n175 = event-data() -> ("NewVal"=w709:bool)  [unwired: 1 in, 5 out]
        n176 = call "Source Output Enable.vi"("Output (Off)"=w709, "error in (no error)"=w714, "Channel (Channel A)"=Channel."Channel B", "Node In"=w712, "VISA resource name"=w711) -> ("error out"=w708:errorcluster, "Node Out"=w707:string, "VISA resource name out"=w713:refnum<visa-resource-name>)  [unwired: 3 in, 1 out]
      }
      event "RESTART": Value Change {
        n177 = event-data() -> ("NewVal"=w719:bool)  [unwired: 1 in, 5 out]
        n178 = case shown="True" w719 {
          tunnel: w721 -> [w730 w740]
          tunnel: w720 -> [w729 w741]
          tunnel: [w730 w739] -> w722
          tunnel: [w729 w738] -> w723
          tunnel: [w728 w734] -> w718
          tunnel: [w727 w733] -> w717
          tunnel: w716 -> [w728 w732]
          tunnel: w715 -> [w727 w731]
          frame False {
          }
          frame True {
            n179 = call "DAQmx Stop Task.vi"("task/channels in"=w740, "error in"=w741) -> ("task out"=w737:refnum<k21>, "error out"=w742:errorcluster)  [unwired: 12 in]
            n180 = call "DAQmx Stop Task.vi"("task/channels in"=w732, "error in"=w731) -> ("task out"=w735:refnum<k21>, "error out"=w736:errorcluster)  [unwired: 12 in]
            n181 = local write "RESTART"(FALSE ("RESTART")) -> ()
            n182 = call "DAQmx Start Task.vi"("task/channels in"=w737, "error in"=w742) -> ("task out"=w739:refnum<k21>, "error out"=w738:errorcluster)  [unwired: 12 in]
            n183 = call "DAQmx Start Task.vi"("task/channels in"=w735, "error in"=w736) -> ("task out"=w734:refnum<k21>, "error out"=w733:errorcluster)  [unwired: 12 in]
          }
        }
      }
    }
    n184 = Subtract(x=w514, y=w516) -> (x-y=w515:dbl)
    n185 = Subtract(x=w530, y=w534) -> (x-y=w533:dbl)
    n186 = Less?(x=w552, y=15.0) -> (x < y?=w508:bool)
    n187 = And(x=w507, y=w508) -> (x .and. y?=w506:bool)
    n188 = Divide(x=w515, y=w499) -> (x/y=→"Rate (Hz)":dbl)
    n189 = Divide(x=w533, y=w499) -> (x/y=→"Rate (Hz)":dbl)
    n190 = case shown="True" w506 {
      tunnel: [FALSE ("RUN/STOP") TRUE ("RUN/STOP")] -> w511
      frame False {
      }
      frame True {
      }
    }
    n191 = property on="READY" class="Bool (strict)"() -> ("Value"=w513:bool)  [unwired: 2 in, 2 out]
    n192 = Equal?(x=w513, y=w511) -> (x = y?=w512:bool)
    n193 = case shown="False" w512 {
      tunnel: w511 -> [w590 _]
      frame False {
        n194 = property on="READY" class="Bool (strict)"("Val(Sgnl)"=w590) -> ()  [unwired: 2 in, 2 out]
      }
      frame True {
      }
    }
    n195 = local read "Kill Switch"() -> (w535:bool)
  }
  n196 = while {
    stop <- w745 stop-if-true
    n197 = event shown="[1] \"COOLDOWN\": Value Change" {
      selector: _ -> [_ _]
      dyn-events: _ -> [_ _]
      timeout: 500 -> [_ _]
      event Timeout {
        n198 = event-data() -> ()  [unwired: 1 in, 3 out]
      }
      event "COOLDOWN": Value Change {
        n199 = event-data() -> ("NewVal"=w746:bool)  [unwired: 1 in, 5 out]
        n200 = case shown="True" w746 {
          frame False {
          }
          frame True {
            n201 = flat-sequence {
              frame #0 {
                n202 = property on="Percent Open" class="DigNum (strict)"("Val(Sgnl)"=100 ("Percent Open")) -> ()  [unwired: 2 in, 2 out]
              }
              frame #1 {
                n203 = while {
                  i -> [w751]
                  stop <- w748 stop-if-true
                  n204 = Greater Than 0?(x=w751) -> (x > 0?=w750:bool)
                  n205 = case shown="True" w750 {
                    tunnel: [FALSE ("Motor free") w753] -> w748
                    frame False {
                    }
                    frame True {
                      n206 = local read "Motor free"() -> (w753:bool)
                    }
                  }
                  n207 = Wait (ms)(milliseconds to wait=u32 50) -> ()  [unwired: 1 out]
                }
              }
              frame #2 {
                n208 = property on="Sample Space Pump" class="Bool (strict)"("Val(Sgnl)"=FALSE ("Sample Space Pump")) -> ()  [unwired: 2 in, 2 out]
                n209 = Wait (ms)(milliseconds to wait=u32 100) -> ()  [unwired: 1 out]
              }
              frame #3 {
                n210 = property on="Siphon Pump" class="Bool (strict)"("Val(Sgnl)"=TRUE ("Siphon Pump")) -> ()  [unwired: 2 in, 2 out]
                n211 = Wait (ms)(milliseconds to wait=u32 100) -> ()  [unwired: 1 out]
              }
              frame #4 {
                n212 = while {
                  stop <- w761 stop-if-true
                  n213 = local read "Kill Switch"() -> (w764:bool)
                  n214 = local read "COOLDOWN"() -> (w759:bool)
                  n215 = property on="Cryostat Temp (K)" class="DigNum (strict)"() -> ("Value"=w766:dbl)  [unwired: 2 in, 2 out]
                  n216 = Not(x=w759) -> (.not. x?=w758:bool)
                  n217 = Less?(x=w766, y=3.8) -> (x < y?=w763:bool)
                  n218 = Or(x=w764, y=w763) -> (x .or. y?=w760:bool)
                  n219 = Or(x=w760, y=w758) -> (x .or. y?=w761:bool)
                  n220 = Wait (ms)(milliseconds to wait=u32 1000) -> ()  [unwired: 1 out]
                }
              }
              frame #5 {
                n221 = while {
                  i -> [w769]
                  stop <- w768 stop-if-true
                  n222 = local read "COOLDOWN"() -> (w774:bool)
                  n223 = local read "Kill Switch"() -> (w771:bool)
                  n224 = Greater?(x=w769, y="Time (s)") -> (0:w770:bool)
                  n225 = Wait (ms)(milliseconds to wait=u32 1000) -> ()  [unwired: 1 out]
                  n226 = Not(x=w774) -> (.not. x?=w773:bool)
                  n227 = Or(x=w770, y=w771) -> (x .or. y?=w772:bool)
                  n228 = Or(x=w772, y=w773) -> (x .or. y?=w768:bool)
                }
              }
              frame #6 {
                n229 = property on="Percent Open" class="DigNum (strict)"("Val(Sgnl)"=0 ("Percent Open")) -> ()  [unwired: 2 in, 2 out]
              }
              frame #7 {
                n230 = while {
                  i -> [w780]
                  stop <- w777 stop-if-true
                  n231 = Greater Than 0?(x=w780) -> (x > 0?=w779:bool)
                  n232 = case shown="True" w779 {
                    tunnel: [FALSE ("Motor free") w782] -> w777
                    frame False {
                    }
                    frame True {
                      n233 = local read "Motor free"() -> (w782:bool)
                    }
                  }
                  n234 = Wait (ms)(milliseconds to wait=u32 50) -> ()  [unwired: 1 out]
                }
              }
              frame #8 {
                n235 = property on="Sample Space Pump" class="Bool (strict)"("Val(Sgnl)"=TRUE ("Sample Space Pump")) -> ()  [unwired: 2 in, 2 out]
                n236 = Wait (ms)(milliseconds to wait=u32 100) -> ()  [unwired: 1 out]
              }
              frame #9 {
                n237 = property on="Siphon Pump" class="Bool (strict)"("Val(Sgnl)"=FALSE ("Siphon Pump")) -> ()  [unwired: 2 in, 2 out]
                n238 = Wait (ms)(milliseconds to wait=u32 100) -> ()  [unwired: 1 out]
              }
              frame #10 {
                n239 = property on="COOLDOWN" class="Bool (strict)"("Val(Sgnl)"=FALSE ("COOLDOWN")) -> ()  [unwired: 2 in, 2 out]
              }
            }
          }
        }
      }
    }
    n240 = local read "Kill Switch"() -> (w745:bool)
  }
  n241 = while {
    shift-right: [w789] -> w55
    shift-left: w57 -> [w790]
    shift-right: [w788] -> w54
    shift-left: w56 -> [w791]
    stop <- w793 stop-if-true
    n242 = event shown="[0] \"READY\", \"SCRIPTING\": Value Change" {
      selector: _ -> [_ _]
      dyn-events: _ -> [_ _]
      timeout: 500 -> [_ _]
      tunnel: w791 -> [w797 w1272]
      tunnel: w790 -> [w798 w1273]
      tunnel: [w796 w1273] -> w789
      tunnel: [w795 w1272] -> w788
      event "READY", "SCRIPTING": Value Change {
        n243 = event-data() -> ()  [unwired: 1 in, 7 out]
        n244 = case shown="True" "SCRIPTING" {
          tunnel: w798 -> [w800 w804]
          tunnel: w797 -> [w799 w803]
          tunnel: [w800 w801] -> w796
          tunnel: [w799 w802] -> w795
          frame False {
          }
          frame True {
            n245 = local read "Script\n#"() -> (w806:i32)
            n246 = Not Equal To 0?(x=w806) -> (x != 0?=w805:bool)
            n247 = case shown="False" w805 {
              tunnel: w804 -> [w812 w996]
              tunnel: w803 -> [w813 w997]
              tunnel: [w807 w994] -> w802
              tunnel: [w808 w995] -> w801
              frame False {
                n248 = call "GetManualCommands.vi"("Manual Script Entry (0)"="Manual Script Entry (0)") -> ("Commands"=w820:string[])  [unwired: 10 in]
                n249 = Array Size(array=w820) -> (size(s)=w816:i32)
                n250 = for {
                  tunnel: w820 -> [w852] mode=indexing
                  tunnel: [w847] -> w819
                  tunnel: [w846] -> w814
                  i -> [w847]
                  stop <- w849 stop-if-true
                  n251 = Match Pattern(string=w852, regular expression="[a-z]+") -> (match substring=w845:string, after substring=w844:string)  [unwired: 1 in, 2 out]
                  n252 = call "Trim Whitespace.vi"("string"=w844) -> ("trimmed string"=w851:string)  [unwired: 1 in]
                  n253 = Concatenate Strings(w845, w844) -> (w843:string)
                  n254 = case shown="\"False\", Default" w845 {
                    tunnel: w851 -> [_ w865 w884 w899 w906 w924 w942 w971]
                    tunnel: [TRUE ("Top Coil") w864 w881 FALSE ("Top Coil") w903 w921 w941 w970] -> w848
                    tunnel: w847 -> [w857 w863 w883 _ w905 w923 w940 w969]
                    tunnel: u32 0 ("Script Number") -> [w856 w862 w882 _ w904 w922 w939 w968]
                    tunnel: [w855 w860 w879 "" ("Error String") w901 w920 w937 w966] -> w846
                    tunnel: w843 -> [w854 w859 w878 _ w900 w919 w936 w965]
                    frame "False", Default {
                      n255 = call "ErrorHandling.vi"("Bad Command"=w854, "Line #"=w857, "Script #"=w856) -> ("Error String"=w855:string)  [unwired: 8 in]
                    }
                    frame "data" {
                      n256 = case shown="\"False\", Default" w865 {
                        tunnel: [FALSE ("DATA") TRUE ("DATA") FALSE ("DATA")] -> w861
                        tunnel: [TRUE ("Top Coil") FALSE ("Top Coil") FALSE ("Top Coil")] -> w864
                        tunnel: w863 -> [w868 _ _]
                        tunnel: w862 -> [w869 _ _]
                        tunnel: [w867 "" ("Error String") "" ("Error String")] -> w860
                        tunnel: w859 -> [w866 _ _]
                        frame "False", Default {
                          n257 = call "ErrorHandling.vi"("Bad Command"=w866, "Line #"=w868, "Script #"=w869) -> ("Error String"=w867:string)  [unwired: 8 in]
                        }
                        frame "on" {
                        }
                        frame "off" {
                        }
                      }
                      n258 = property on="DATA" class="Bool (strict)"("Val(Sgnl)"=w861) -> ()  [unwired: 2 in, 2 out]
                    }
                    frame "pulse" {
                      n259 = case shown="\"False\", Default" w884 {
                        tunnel: [FALSE ("Top Coil") TRUE ("Top Coil") w895] -> w880
                        tunnel: [TRUE FALSE w895] -> w881
                        tunnel: w883 -> [w888 _ _]
                        tunnel: w882 -> [w887 _ _]
                        tunnel: [w886 "" ""] -> w879
                        tunnel: w878 -> [w885 _ _]
                        frame "False", Default {
                          n260 = call "ErrorHandling.vi"("Bad Command"=w885, "Line #"=w888, "Script #"=w887) -> ("Error String"=w886:string)  [unwired: 8 in]
                        }
                        frame "on" {
                        }
                        frame "off" {
                          w895 = FALSE ("Top Coil")
                        }
                      }
                      n261 = property on="RUN/STOP" class="Bool (strict)"("Val(Sgnl)"=w880) -> ()  [unwired: 2 in, 2 out]
                    }
                    frame "wait" {
                      n262 = Decimal String To Number(string=w899) -> (number=w898:i32)  [unwired: 2 in, 1 out]
                      n263 = Wait (ms)(milliseconds to wait=w898) -> ()  [unwired: 1 out]
                    }
                    frame "neutron" {
                      n264 = case shown="\"False\", Default" w906 {
                        tunnel: w905 -> [w912 _ _]
                        tunnel: w904 -> [w911 _ _]
                        tunnel: [TRUE ("Top Coil") FALSE ("Top Coil") w917] -> w903
                        tunnel: [FALSE ("Neutron Shutter") TRUE ("Neutron Shutter") w917] -> w902
                        tunnel: [w908 "" ("Error String") "" ("Error String")] -> w901
                        tunnel: w900 -> [w907 _ _]
                        frame "False", Default {
                          n265 = call "ErrorHandling.vi"("Bad Command"=w907, "Line #"=w912, "Script #"=w911) -> ("Error String"=w908:string)  [unwired: 8 in]
                        }
                        frame "on" {
                        }
                        frame "off" {
                          w917 = FALSE ("Neutron Shutter")
                        }
                      }
                      n266 = property on="Neutron Shutter" class="Bool (strict)"("Val(Sgnl)"=w902) -> ()  [unwired: 2 in, 2 out]
                    }
                    frame "shutter" {
                      n267 = case shown="\"False\", Default" w924 {
                        tunnel: w923 -> [w930 _ _]
                        tunnel: w922 -> [w929 _ _]
                        tunnel: [TRUE ("Top Coil") FALSE ("Top Coil") w935] -> w921
                        tunnel: [FALSE ("Neutron Shutter") TRUE ("Neutron Shutter") w935] -> w918
                        tunnel: [w926 "" ("Error String") "" ("Error String")] -> w920
                        tunnel: w919 -> [w925 _ _]
                        frame "False", Default {
                          n268 = call "ErrorHandling.vi"("Bad Command"=w925, "Line #"=w930, "Script #"=w929) -> ("Error String"=w926:string)  [unwired: 8 in]
                        }
                        frame "on" {
                        }
                        frame "off" {
                          w935 = FALSE ("Neutron Shutter")
                        }
                      }
                      n269 = property on="Enable" class="Bool (strict)"("Val(Sgnl)"=w918) -> ()  [unwired: 2 in, 2 out]
                    }
                    frame "coila" {
                      n270 = case shown="\"False\", Default" w942 {
                        selector: w942 -> [w949 _]
                        tunnel: [w951 w964] -> w938
                        tunnel: [w950 w964] -> w941
                        tunnel: w940 -> [w946 _]
                        tunnel: w939 -> [w945 _]
                        tunnel: [w944 "" ("Error String")] -> w937
                        tunnel: w936 -> [w943 _]
                        frame "False", Default {
                          n271 = Match Pattern(string=w949, regular expression="[^0-9.]") -> (offset past match=w947:i32)  [unwired: 1 in, 3 out]
                          n272 = case shown="0, Default" w947 {
                            tunnel: [FALSE ("Top Coil") TRUE ("Top Coil")] -> w951
                            tunnel: [TRUE FALSE] -> w950
                            tunnel: w949 -> [_ w960]
                            tunnel: w946 -> [w955 _]
                            tunnel: w945 -> [w954 _]
                            tunnel: [w953 ""] -> w944
                            tunnel: w943 -> [w952 _]
                            frame 0, Default {
                              n273 = call "ErrorHandling.vi"("Bad Command"=w952, "Line #"=w955, "Script #"=w954) -> ("Error String"=w953:string)  [unwired: 8 in]
                            }
                            frame -1 {
                              n274 = Fract/Exp String To Number(string=w960) -> (number=w959:dbl)  [unwired: 3 in, 1 out]
                              n275 = property on="Top Coil (mA)" class="DigNum (strict)"("Val(Sgnl)"=w959) -> ()  [unwired: 2 in, 2 out]
                            }
                          }
                        }
                        frame "off" {
                          w964 = FALSE ("Top Coil")
                        }
                      }
                      n276 = property on="Top Coil" class="Bool (strict)"("Val(Sgnl)"=w938) -> ()  [unwired: 2 in, 2 out]
                    }
                    frame "coilb" {
                      n277 = case shown="\"False\", Default" w971 {
                        selector: w971 -> [w978 _]
                        tunnel: [w977 w993] -> w967
                        tunnel: [w976 w993] -> w970
                        tunnel: w969 -> [w975 _]
                        tunnel: w968 -> [w974 _]
                        tunnel: [w973 ""] -> w966
                        tunnel: w965 -> [w972 _]
                        frame "False", Default {
                          n278 = Match Pattern(string=w978, regular expression="[^0-9.]") -> (offset past match=w979:i32)  [unwired: 1 in, 3 out]
                          n279 = case shown="0, Default" w979 {
                            tunnel: w978 -> [_ w991]
                            tunnel: [FALSE TRUE] -> w977
                            tunnel: [TRUE FALSE] -> w976
                            tunnel: w975 -> [w984 _]
                            tunnel: w974 -> [w983 _]
                            tunnel: [w982 ""] -> w973
                            tunnel: w972 -> [w981 _]
                            frame 0, Default {
                              n280 = call "ErrorHandling.vi"("Bad Command"=w981, "Line #"=w984, "Script #"=w983) -> ("Error String"=w982:string)  [unwired: 8 in]
                            }
                            frame -1 {
                              n281 = Fract/Exp String To Number(string=w991) -> (number=w988:dbl)  [unwired: 3 in, 1 out]
                              n282 = property on="Bottom Coil (mA)" class="DigNum (strict)"("Val(Sgnl)"=w988) -> ()  [unwired: 2 in, 2 out]
                            }
                          }
                        }
                        frame "off" {
                          w993 = FALSE
                        }
                      }
                      n283 = property on="Bottom Coil" class="Bool (strict)"("Val(Sgnl)"=w967) -> ()  [unwired: 2 in, 2 out]
                    }
                  }
                  n284 = local read "Kill Switch"() -> (w842:bool)
                  n285 = Or(x=w848, y=w842) -> (x .or. y?=w849:bool)
                }
                n286 = Decrement(x=w816) -> (x-1=w818:i32)
                n287 = Equal?(x=w819, y=w818) -> (x = y?=w817:bool)
                n288 = case shown="False" w817 {
                  tunnel: [w836 w839] -> w815
                  tunnel: w814 -> [w834 _]
                  tunnel: [w832 w838] -> w810
                  frame False {
                    w831 = FALSE ("status")
                    n289 = property on="Bottom Coil" class="Bool (strict)"("Val(Sgnl)"=w831) -> ()  [unwired: 2 in, 2 out]
                    n290 = property on="Neutron Shutter" class="Bool (strict)"("Val(Sgnl)"=w831) -> ()  [unwired: 2 in, 2 out]
                    n291 = property on="Top Coil" class="Bool (strict)"("Val(Sgnl)"=w831) -> ()  [unwired: 2 in, 2 out]
                    n292 = property on="Enable" class="Bool (strict)"("Val(Sgnl)"=w831) -> ()  [unwired: 2 in, 2 out]
                    n293 = property on="RUN/STOP" class="Bool (strict)"("Val(Sgnl)"=w831) -> ()  [unwired: 2 in, 2 out]
                    n294 = property on="DATA" class="Bool (strict)"("Val(Sgnl)"=w831) -> ()  [unwired: 2 in, 2 out]
                    n295 = Concatenate Strings("Manual test failed!" ("Description"), "\r\n", w834) -> (w832:string)
                    n296 = Bundle("status"=w831, "code"=1017, w832) -> (w836:cluster{"status":bool, "code":i32, string})  [unwired: 1 in]
                  }
                  frame True {
                    w838 = "Manual test successful!" ("Description")
                    n297 = Bundle("status"=FALSE, "code"=0, "Description"=w838) -> (w839:T2)  [unwired: 1 in]
                  }
                }
                n298 = flat-sequence {
                  tunnel: w815 -> [w828]
                  tunnel: w813 -> [w824]
                  tunnel: w812 -> [w827]
                  tunnel: "Manual Script Entry (0)" -> [w826]
                  tunnel: w810 -> [w825]
                  tunnel: [w823] -> w809
                  tunnel: [w822] -> w807
                  tunnel: w809 -> [w830]
                  tunnel: [w830] -> w808
                  frame #0 {
                    n299 = local write "Scripting \nError"(w828) -> ()
                    n300 = local read "Timestamp"() -> (w821:string)
                    n301 = call "WriteResults_Manual.vi"("Timestamp"=w821, "error in"=w824, "Result"=w825, "Commands"=w826, "refnum in"=w827) -> ("error out"=w822:errorcluster, "refnum out"=w823:refnum<file>)  [unwired: 5 in]
                  }
                  frame #1 {
                    n302 = property on="SCRIPTING" class="Bool (strict)"("Val(Sgnl)"=FALSE ("Value (Signaling)")) -> ()  [unwired: 2 in, 2 out]
                  }
                }
              }
              frame True {
                n303 = while {
                  tunnel: w997 -> [w1003]
                  tunnel: w996 -> [w1002]
                  tunnel: [w1001] -> w995
                  tunnel: [w999] -> w994
                  stop <- w998 stop-if-true
                  n304 = local read "Script\n#"() -> (w1005:i32)
                  n305 = call "GetCommands.vi"("Script Number"=w1005) -> ("Script Exists"=w1006:bool, "Commands"=w1007:string[], "Camera Settings"=w1008:dbl[], "Data Interval (s)"=w1004:dbl)  [unwired: 5 in]
                  n306 = case shown="True" w1006 {
                    tunnel: w1008 -> [_ w1042]
                    tunnel: w1007 -> [_ w1040]
                    tunnel: w1005 -> [w1025 w1038]
                    tunnel: w1004 -> [_ w1037]
                    tunnel: w1003 -> [w1019 w1035]
                    tunnel: w1002 -> [w1020 w1034]
                    tunnel: [w1018 w1033] -> w1001
                    tunnel: [w1017 w1032] -> w1000
                    frame False {
                      n307 = Number To Decimal String(number=w1025) -> (decimal integer string=w1024:string)  [unwired: 1 in]
                      n308 = Concatenate Strings("Script" ("string"), w1024, " does not exist." ("string")) -> (w1021:string)
                      n309 = Bundle("status"=FALSE, "code"=1017, w1021) -> (w1026:cluster{"status":bool, "code":i32, string})  [unwired: 1 in]
                      n310 = Get Date/Time In Seconds() -> (seconds since 1Jan1904=w1016:timestamp)
                      n311 = Format Date/Time String(time format string (%c)="%H:%M:%S", seconds (now)=w1016) -> (date/time string=w1014:string)  [unwired: 1 in]
                      n312 = local write "Scripting \nError"(w1026) -> ()
                      n313 = call "WriteResults_Script.vi"("Timestamp"=w1014, "error in"=w1019, "Result"=w1021, "refnum in"=w1020) -> ("error out"=w1017:errorcluster, "refnum out"=w1018:refnum<file>)  [unwired: 6 in]
                      n314 = property on="SCRIPTING" class="Bool (strict)"("Val(Sgnl)"=FALSE ("Value (Signaling)")) -> ()  [unwired: 2 in, 2 out]
                    }
                    frame True {
                      n315 = flat-sequence {
                        tunnel: u32 100 ("milliseconds to wait") -> [w1053]
                        tunnel: w1042 -> [w1054]
                        tunnel: [w1054] -> w1031
                        tunnel: [w1053] -> w1030
                        tunnel: w1037 -> [w1052]
                        tunnel: w1031 -> [w1058]
                        tunnel: [w1058] -> w1051
                        tunnel: w1030 -> [w1057]
                        tunnel: [w1057] -> w1050
                        tunnel: w1051 -> [w1063]
                        tunnel: [w1063] -> w1049
                        tunnel: w1050 -> [w1062]
                        tunnel: [w1062] -> w1048
                        tunnel: w1049 -> [w1067]
                        tunnel: [w1067] -> w1047
                        tunnel: w1048 -> [w1066]
                        tunnel: [w1066] -> w1046
                        tunnel: w1047 -> [w1071]
                        tunnel: [w1071] -> w1045
                        tunnel: w1046 -> [w1070]
                        tunnel: [w1070] -> w1044
                        tunnel: w1045 -> [w1076]
                        tunnel: w1044 -> [w1075]
                        tunnel: w1040 -> [w1081]
                        tunnel: w1038 -> [w1080]
                        tunnel: [w1079] -> w1043
                        tunnel: [w1078] -> w1036
                        tunnel: w1039 -> [w1244]
                        tunnel: w1043 -> [w1245]
                        tunnel: w1038 -> [w1234]
                        tunnel: w1036 -> [w1241]
                        tunnel: w1035 -> [w1238]
                        tunnel: w1034 -> [w1239]
                        tunnel: [w1237] -> w1033
                        tunnel: [w1236] -> w1032
                        frame #0 {
                          n316 = property on="Data Interval (s)" class="DigNum (strict)"("Val(Sgnl)"=w1052) -> ()  [unwired: 2 in, 2 out]
                        }
                        frame #1 {
                          n317 = Index Array(array=w1058, index=0) -> (element=w1056:dbl)
                          n318 = To Unsigned Word Integer(number=w1056) -> (unsigned 16bit integer=w1055:u16)
                          n319 = local write "MODE"(w1055) -> ()
                        }
                        frame #2 {
                          n320 = Index Array(array=w1063, index=1) -> (element=w1061:dbl)
                          n321 = To Unsigned Word Integer(number=w1061) -> (unsigned 16bit integer=w1060:u16)
                          n322 = local write "BIN"(w1060) -> ()
                        }
                        frame #3 {
                          n323 = Index Array(array=w1067, index=2) -> (element=w1065:dbl)
                          n324 = local write "On CCD Acc."(w1065) -> ()
                        }
                        frame #4 {
                          n325 = Index Array(array=w1071, index=3) -> (element=w1069:dbl)
                          n326 = property on="# Frames" class="DigNum (strict)"("Val(Sgnl)"=w1069) -> ()  [unwired: 2 in, 2 out]
                          n327 = Wait (ms)(milliseconds to wait=w1070) -> ()  [unwired: 1 out]
                        }
                        frame #5 {
                          n328 = Index Array(array=w1076, index=4) -> (element=w1074:dbl)
                          n329 = To Unsigned Word Integer(number=w1074) -> (unsigned 16bit integer=w1073:u16)
                          n330 = property on="Shutter Mode" class="Ring (strict)"("Val(Sgnl)"=w1073) -> ()  [unwired: 2 in, 2 out]
                          n331 = Wait (ms)(milliseconds to wait=w1075) -> ()  [unwired: 1 out]
                        }
                        frame #6 {
                          n332 = for {
                            tunnel: w1081 -> [w1093] mode=indexing
                            tunnel: w1080 -> [w1090]
                            tunnel: [w1087] -> w1079
                            tunnel: [w1086] -> w1078
                            i -> [w1087]
                            stop <- w1082 stop-if-true
                            n333 = Match Pattern(string=w1093, regular expression="[a-z]+") -> (match substring=w1085:string, after substring=w1084:string)  [unwired: 1 in, 2 out]
                            n334 = call "Trim Whitespace.vi"("string"=w1084) -> ("trimmed string"=w1091:string)  [unwired: 1 in]
                            n335 = Concatenate Strings(w1085, w1084) -> (w1083:string)
                            n336 = case shown="\"shutter\"" w1085 {
                              tunnel: w1091 -> [_ w1105 w1124 w1139 w1146 w1164 w1182 w1211]
                              tunnel: [TRUE ("Top Coil") w1104 w1121 FALSE ("Top Coil") w1143 w1161 w1181 w1210] -> w1089
                              tunnel: w1087 -> [w1097 w1103 w1123 _ w1145 w1163 w1180 w1209]
                              tunnel: w1090 -> [w1096 w1102 w1122 _ w1144 w1162 w1179 w1208]
                              tunnel: [w1094 w1100 w1119 "" ("Error String") w1141 w1160 w1177 w1206] -> w1086
                              tunnel: w1083 -> [w1095 w1099 w1118 _ w1140 w1159 w1176 w1205]
                              frame "False", Default {
                                n337 = call "ErrorHandling.vi"("Bad Command"=w1095, "Line #"=w1097, "Script #"=w1096) -> ("Error String"=w1094:string)  [unwired: 8 in]
                              }
                              frame "data" {
                                n338 = case shown="\"False\", Default" w1105 {
                                tunnel: [FALSE ("DATA") TRUE ("DATA") FALSE ("DATA")] -> w1101
                                tunnel: [TRUE ("Top Coil") FALSE ("Top Coil") FALSE ("Top Coil")] -> w1104
                                tunnel: w1103 -> [w1108 _ _]
                                tunnel: w1102 -> [w1109 _ _]
                                tunnel: [w1107 "" ""] -> w1100
                                tunnel: w1099 -> [w1106 _ _]
                                frame "False", Default {
                                n339 = call "ErrorHandling.vi"("Bad Command"=w1106, "Line #"=w1108, "Script #"=w1109) -> ("Error String"=w1107:string)  [unwired: 8 in]
                                }
                                frame "on" {
                                }
                                frame "off" {
                                }
                                }
                                n340 = property on="DATA" class="Bool (strict)"("Val(Sgnl)"=w1101) -> ()  [unwired: 2 in, 2 out]
                              }
                              frame "pulse" {
                                n341 = case shown="\"False\", Default" w1124 {
                                tunnel: [FALSE ("Top Coil") TRUE ("Top Coil") w1135] -> w1120
                                tunnel: [TRUE FALSE w1135] -> w1121
                                tunnel: w1123 -> [w1128 _ _]
                                tunnel: w1122 -> [w1127 _ _]
                                tunnel: [w1126 "" ("Error String") ""] -> w1119
                                tunnel: w1118 -> [w1125 _ _]
                                frame "False", Default {
                                n342 = call "ErrorHandling.vi"("Bad Command"=w1125, "Line #"=w1128, "Script #"=w1127) -> ("Error String"=w1126:string)  [unwired: 8 in]
                                }
                                frame "on" {
                                }
                                frame "off" {
                                w1135 = FALSE ("Top Coil")
                                }
                                }
                                n343 = property on="RUN/STOP" class="Bool (strict)"("Val(Sgnl)"=w1120) -> ()  [unwired: 2 in, 2 out]
                              }
                              frame "wait" {
                                n344 = Decimal String To Number(string=w1139) -> (number=w1138:i32)  [unwired: 2 in, 1 out]
                                n345 = Wait (ms)(milliseconds to wait=w1138) -> ()  [unwired: 1 out]
                              }
                              frame "neutron" {
                                n346 = case shown="\"on\"" w1146 {
                                tunnel: w1145 -> [w1152 _ _]
                                tunnel: w1144 -> [w1151 _ _]
                                tunnel: [TRUE ("Top Coil") FALSE ("Top Coil") w1157] -> w1143
                                tunnel: [FALSE ("Neutron Shutter") TRUE ("Neutron Shutter") w1157] -> w1142
                                tunnel: [w1148 "" ""] -> w1141
                                tunnel: w1140 -> [w1147 _ _]
                                frame "False", Default {
                                n347 = call "ErrorHandling.vi"("Bad Command"=w1147, "Line #"=w1152, "Script #"=w1151) -> ("Error String"=w1148:string)  [unwired: 8 in]
                                }
                                frame "on" {
                                }
                                frame "off" {
                                w1157 = FALSE ("Neutron Shutter")
                                }
                                }
                                n348 = property on="Neutron Shutter" class="Bool (strict)"("Val(Sgnl)"=w1142) -> ()  [unwired: 2 in, 2 out]
                              }
                              frame "shutter" {
                                n349 = case shown="\"off\"" w1164 {
                                tunnel: w1163 -> [w1170 _ _]
                                tunnel: w1162 -> [w1169 _ _]
                                tunnel: [TRUE ("Top Coil") FALSE ("Top Coil") w1175] -> w1161
                                tunnel: [FALSE ("Neutron Shutter") TRUE ("Neutron Shutter") w1175] -> w1158
                                tunnel: [w1166 "" ""] -> w1160
                                tunnel: w1159 -> [w1165 _ _]
                                frame "False", Default {
                                n350 = call "ErrorHandling.vi"("Bad Command"=w1165, "Line #"=w1170, "Script #"=w1169) -> ("Error String"=w1166:string)  [unwired: 8 in]
                                }
                                frame "on" {
                                }
                                frame "off" {
                                w1175 = FALSE ("Neutron Shutter")
                                }
                                }
                                n351 = property on="Enable" class="Bool (strict)"("Val(Sgnl)"=w1158) -> ()  [unwired: 2 in, 2 out]
                              }
                              frame "coila" {
                                n352 = case shown="\"False\", Default" w1182 {
                                selector: w1182 -> [w1189 _]
                                tunnel: [w1191 w1204] -> w1178
                                tunnel: [w1190 w1204] -> w1181
                                tunnel: w1180 -> [w1186 _]
                                tunnel: w1179 -> [w1185 _]
                                tunnel: [w1184 ""] -> w1177
                                tunnel: w1176 -> [w1183 _]
                                frame "False", Default {
                                n353 = Match Pattern(string=w1189, regular expression="[^0-9.]") -> (offset past match=w1187:i32)  [unwired: 1 in, 3 out]
                                n354 = case shown="-1" w1187 {
                                tunnel: [FALSE ("Top Coil") TRUE ("Top Coil")] -> w1191
                                tunnel: [TRUE FALSE] -> w1190
                                tunnel: w1189 -> [_ w1200]
                                tunnel: w1186 -> [w1195 _]
                                tunnel: w1185 -> [w1194 _]
                                tunnel: [w1193 ""] -> w1184
                                tunnel: w1183 -> [w1192 _]
                                frame 0, Default {
                                n355 = call "ErrorHandling.vi"("Bad Command"=w1192, "Line #"=w1195, "Script #"=w1194) -> ("Error String"=w1193:string)  [unwired: 8 in]
                                }
                                frame -1 {
                                n356 = Fract/Exp String To Number(string=w1200) -> (number=w1199:dbl)  [unwired: 3 in, 1 out]
                                n357 = property on="Top Coil (mA)" class="DigNum (strict)"("Val(Sgnl)"=w1199) -> ()  [unwired: 2 in, 2 out]
                                }
                                }
                                }
                                frame "off" {
                                w1204 = FALSE ("Top Coil")
                                }
                                }
                                n358 = property on="Top Coil" class="Bool (strict)"("Val(Sgnl)"=w1178) -> ()  [unwired: 2 in, 2 out]
                              }
                              frame "coilb" {
                                n359 = case shown="\"off\"" w1211 {
                                selector: w1211 -> [w1218 _]
                                tunnel: [w1217 w1233] -> w1207
                                tunnel: [w1216 w1233] -> w1210
                                tunnel: w1209 -> [w1215 _]
                                tunnel: w1208 -> [w1214 _]
                                tunnel: [w1213 "" ("Error String")] -> w1206
                                tunnel: w1205 -> [w1212 _]
                                frame "False", Default {
                                n360 = Match Pattern(string=w1218, regular expression="[^0-9.]") -> (offset past match=w1219:i32)  [unwired: 1 in, 3 out]
                                n361 = case shown="-1" w1219 {
                                tunnel: w1218 -> [_ w1231]
                                tunnel: [FALSE TRUE] -> w1217
                                tunnel: [TRUE FALSE] -> w1216
                                tunnel: w1215 -> [w1224 _]
                                tunnel: w1214 -> [w1223 _]
                                tunnel: [w1222 ""] -> w1213
                                tunnel: w1212 -> [w1221 _]
                                frame 0, Default {
                                n362 = call "ErrorHandling.vi"("Bad Command"=w1221, "Line #"=w1224, "Script #"=w1223) -> ("Error String"=w1222:string)  [unwired: 8 in]
                                }
                                frame -1 {
                                n363 = Fract/Exp String To Number(string=w1231) -> (number=w1228:dbl)  [unwired: 3 in, 1 out]
                                n364 = property on="Bottom Coil (mA)" class="DigNum (strict)"("Val(Sgnl)"=w1228) -> ()  [unwired: 2 in, 2 out]
                                }
                                }
                                }
                                frame "off" {
                                w1233 = FALSE
                                }
                                }
                                n365 = property on="Bottom Coil" class="Bool (strict)"("Val(Sgnl)"=w1207) -> ()  [unwired: 2 in, 2 out]
                              }
                            }
                            n366 = local read "Kill Switch"() -> (w1088:bool)
                            n367 = Or(x=w1089, y=w1088) -> (x .or. y?=w1082:bool)
                          }
                        }
                        frame #7 {
                          n368 = Decrement(x=w1244) -> (x-1=w1243:i32)
                          n369 = Equal?(x=w1245, y=w1243) -> (x = y?=w1246:bool)
                          n370 = case shown="True" w1246 {
                            tunnel: w1234 -> [w1255 w1260]
                            tunnel: [w1254 w1267] -> w1242
                            tunnel: w1241 -> [w1250 _]
                            tunnel: [w1248 w1261] -> w1240
                            frame False {
                              w1247 = FALSE ("Value (Signaling)")
                              n371 = Number To Decimal String(number=w1255) -> (decimal integer string=w1252:string)  [unwired: 1 in]
                              n372 = property on="Top Coil" class="Bool (strict)"("Val(Sgnl)"=w1247) -> ()  [unwired: 2 in, 2 out]
                              n373 = property on="Bottom Coil" class="Bool (strict)"("Val(Sgnl)"=w1247) -> ()  [unwired: 2 in, 2 out]
                              n374 = property on="SCRIPTING" class="Bool (strict)"("Val(Sgnl)"=w1247) -> ()  [unwired: 2 in, 2 out]
                              n375 = property on="Neutron Shutter" class="Bool (strict)"("Val(Sgnl)"=w1247) -> ()  [unwired: 2 in, 2 out]
                              n376 = property on="DATA" class="Bool (strict)"("Val(Sgnl)"=w1247) -> ()  [unwired: 2 in, 2 out]
                              n377 = property on="RUN/STOP" class="Bool (strict)"("Val(Sgnl)"=w1247) -> ()  [unwired: 2 in, 2 out]
                              n378 = Concatenate Strings("Script" ("string"), w1252, " failed!" ("string"), "\r\n", w1250) -> (w1248:string)
                              n379 = Bundle(FALSE, 1017, w1248) -> (w1254:errorcluster)  [unwired: 1 in]
                              n380 = property on="Enable" class="Bool (strict)"("Val(Sgnl)"=w1247) -> ()  [unwired: 2 in, 2 out]
                            }
                            frame True {
                              n381 = Number To Decimal String(number=w1260) -> (decimal integer string=w1263:string)  [unwired: 1 in]
                              n382 = Less?(x=w1260, y="Script\nEnd") -> (x < y?=w1258:bool)
                              n383 = case shown="False" w1258 {
                                tunnel: w1260 -> [_ w1270]
                                frame False {
                                n384 = property on="SCRIPTING" class="Bool (strict)"("Val(Sgnl)"=FALSE ("Value (Signaling)")) -> ()  [unwired: 2 in, 2 out]
                                }
                                frame True {
                                n385 = Increment(x=w1270) -> (x+1=w1271:i32)
                                n386 = property on="Script\n#" class="DigNum (strict)"("Val(Sgnl)"=w1271) -> ()  [unwired: 2 in, 2 out]
                                n387 = Wait (ms)(milliseconds to wait=u32 5000) -> ()  [unwired: 1 out]
                                }
                              }
                              n388 = Concatenate Strings("Script" ("string"), w1263, " successful!" ("string")) -> (w1261:string)
                              n389 = Bundle(FALSE, 0, w1261) -> (w1267:errorcluster)  [unwired: 1 in]
                            }
                          }
                          "Scripting \nError" <- w1242
                          n390 = local read "Timestamp"() -> (w1235:string)
                          n391 = call "WriteResults_Script.vi"("Timestamp"=w1235, "error in"=w1238, "Result"=w1240, "refnum in"=w1239) -> ("error out"=w1236:errorcluster, "refnum out"=w1237:refnum<file>)  [unwired: 6 in]
                        }
                      }
                      n392 = Array Size(array=w1040) -> (size(s)=w1039:i32)
                    }
                  }
                  n393 = flat-sequence {
                    tunnel: w1000 -> [w1011]
                    tunnel: [w1011] -> w999
                    tunnel: [w1010] -> w998
                    frame #0 {
                      n394 = local read "SCRIPTING"() -> (w1012:bool)
                      n395 = local read "Kill Switch"() -> (w1009:bool)
                      n396 = Not(x=w1012) -> (.not. x?=w1013:bool)
                      n397 = Or(x=w1013, y=w1009) -> (x .or. y?=w1010:bool)
                    }
                  }
                }
              }
            }
          }
        }
      }
      event Timeout {
        n398 = event-data() -> ()  [unwired: 1 in, 3 out]
      }
    }
    n399 = local read "Kill Switch"() -> (w793:bool)
  }
  n400 = flat-sequence {
    tunnel: w11 -> [w1275]
    tunnel: [w1275] -> w10
    tunnel: [w1274] -> w9
    frame #0 {
      n401 = local read "LIGHTFIELD"() -> (w1274:bool)
    }
  }
  n402 = call "NeedleValveClose.vi"("error in (no error)"=w112, "VISA resource name"=w113) -> ("error out"=w35:errorcluster, "VISA resource name out"=w37:refnum<visa-resource-name>)  [unwired: 8 in]
  n403 = call "RelayControl.vi"("Neutron Shutter"=w60, "Error In"=w81, "Sample Space Pump"=w60, "Siphon Pump"=w60, "Relay In"=w79) -> ("Error Out"=w80:errorcluster, "Relay Out"=w78:refnum<visa-resource-name>)  [unwired: 5 in]
  n404 = flat-sequence {
    tunnel: [w1277] -> w6
    tunnel: w7 -> [w1277]
    tunnel: [w1276] -> w5
    frame #0 {
      n405 = local read "Enable"() -> (w1276:bool)
    }
  }
  n406 = flat-sequence {
    tunnel: [w1281] -> w74
    tunnel: [w1280] -> w75
    tunnel: w76 -> [w1279]
    tunnel: w77 -> [w1278]
    frame #0 {
      n407 = VISA Write(VISA resource name=w1279, write buffer=":PULSE0:STATE OFF\r\n" ("format string"), error in (no error)=w1278) -> (VISA resource name out=w1280:refnum<visa-resource-name>, error out=w1281:errorcluster)  [unwired: 1 out]
    }
  }
  n408 = VISA Close(VISA resource name=w78, error in (no error)=w80) -> (error out=w73:errorcluster)
  n409 = flat-sequence {
    tunnel: w35 -> [w1283]
    tunnel: [w1283] -> w38
    tunnel: [w1286] -> w36
    tunnel: w38 -> [w1286]
    frame #0 {
      n410 = Wait (ms)(milliseconds to wait=u32 3000) -> ()  [unwired: 1 out]
    }
    frame #1 {
      n411 = local write "Percent Open"(0 ("Percent Open")) -> ()
    }
  }
  n412 = flat-sequence {
    tunnel: w60 -> [w1287]
    tunnel: [w1288] -> w72
    tunnel: w73 -> [w1288]
    frame #0 {
      n413 = local write "Siphon Pump"(w1287) -> ()
      n414 = local write "Sample Space Pump"(w1287) -> ()
      n415 = local write "Neutron Shutter"(w1287) -> ()
    }
  }
  n416 = case shown="False" w5 {
    tunnel: [w1290 w1294] -> w16
    tunnel: [w1289 w1293] -> w15
    tunnel: w14 -> [w1289 w1292]
    tunnel: w6 -> [w1290 w1291]
    frame False {
    }
    frame True {
      n417 = call "ToggleShutter.vi"("error in"=w1291, "VISA resource name"=w1292) -> ("error out"=w1294:errorcluster, "VISA resource name out"=w1293:refnum<visa-resource-name>)  [unwired: 8 in]
    }
  }
  n418 = Equal?(x=w9, y=TRUE) -> (x = y?=w17:bool)
  n419 = call "DAQmx Stop Task.vi"("task/channels in"=w29, "error in"=w28) -> ()  [unwired: 12 in, 2 out]
  n420 = call "DAQmx Stop Task.vi"("task/channels in"=w20, "error in"=w19) -> ()  [unwired: 12 in, 2 out]
  n421 = call "Close.vi"("error in (no error)"=w127, "Mercury Reference"=w126) -> ("error out"=w92:errorcluster)  [unwired: 9 in]
  n422 = case shown="False" w17 {
    tunnel: w18 -> [w1295 w1299]
    tunnel: w10 -> [_ w1298]
    frame False {
      n423 = local write "LightField Error"(w1295) -> ()
    }
    frame True {
      n424 = call "Adv_Deregister_for_Callback.vi"("error in (no error)"=w1299, "LightField Automation in"=w1298) -> ("error out"=w1300:errorcluster, "LightField Automation out"=w1301:refnum<class "LightField Automation.lvclass">)  [unwired: 8 in]
      n425 = call "LFA_Close.vi"("error in (no error)"=w1300, "LightField Automation in"=w1301) -> ("error out"=w1297:errorcluster)  [unwired: 8 in, 1 out]
      n426 = flat-sequence {
        tunnel: w1297 -> [w1303]
        tunnel: [w1303] -> w1296
        frame #0 {
          n427 = local write "LIGHTFIELD"(FALSE ("LIGHTFIELD")) -> ()
        }
      }
      n428 = local write "LightField Error"(w1296) -> ()
    }
  }
  n429 = call "Disconnect From Meter.vi"("Location of FieldMax2Lib.dll in"=w65, "Meter ID in"=w66) -> ()  [unwired: 7 in, 2 out]
  n430 = VISA Close(VISA resource name=w15, error in (no error)=w16) -> (error out=w13:errorcluster)
  n431 = call "KeithleyClose.vi"("Keithley Error In"=w88, "Node In"=w87, "KeithleyVISA In"=w86) -> ("Heater Error"=w85:errorcluster)  [unwired: 8 in]
  n432 = VISA Close(VISA resource name=w116, error in (no error)=w117) -> (error out=→"4He Gauge Error":errorcluster)
  n433 = call "3HeClose.vi"("error in (no error)"=w101, "VISA resource name"=w102) -> ("error out"=→"3He Gauge Error":errorcluster)  [unwired: 9 in]
  n434 = Not Equal?(x=refnum<file> refnum, y=w61) -> (x != y?=w63:bool)
  n435 = VISA Close(VISA resource name=w75, error in (no error)=w74) -> (error out=→"Pulse Generator Error":errorcluster)
  n436 = flat-sequence {
    tunnel: w85 -> [w1305]
    tunnel: [w1305] -> w84
    frame #0 {
      w1304 = FALSE ("Top Coil")
      n437 = local write "Top Coil"(w1304) -> ()
      n438 = local write "Bottom Coil"(w1304) -> ()
    }
  }
  n439 = VISA Close(VISA resource name=w37, error in (no error)=w36) -> (error out=w90:errorcluster)
  n440 = flat-sequence {
    tunnel: w13 -> [w1307]
    tunnel: [w1307] -> w12
    frame #0 {
      n441 = local write "Enable"(FALSE ("Enable")) -> ()
    }
  }
  n442 = case shown="True" w63 {
    tunnel: w62 -> [_ w1310]
    tunnel: w61 -> [_ w1309]
    frame False {
    }
    frame True {
      n443 = Close File(refnum=w1309, error in=w1310) -> (error out=w1308:errorcluster)  [unwired: 1 out]
      n444 = local write "File I/O Error"(w1308) -> ()
    }
  }
  n445 = flat-sequence {
    tunnel: w92 -> [w1315]
    tunnel: [w1315] -> w91
    tunnel: w90 -> [w1314]
    tunnel: [w1314] -> w89
    tunnel: [T2 {"status"=FALSE, "code"=0, "Description"=""} ("Scripting \nError")] -> w59
    tunnel: [w1312] -> w52
    tunnel: w53 -> [w1312]
    frame #0 {
      w1311 = FALSE ("Kill Switch")
      n446 = local write "Kill Switch"(w1311) -> ()
      n447 = local write "READY"(w1311) -> ()
      n448 = local write "LIGHTFIELD"(w1311) -> ()
    }
  }
  n449 = local write "Scripting \nError"(w59) -> ()
  n450 = Close File(refnum=w55, error in=w54) -> (error out=w53:errorcluster)  [unwired: 1 out]
  "Temperature Error" <- w91
  "Heater Error" <- w84
  "Relay Errror" <- w72
  "Zaber Motor Error" <- w89
  "Log Error" <- w52
  "Shutter Error" <- w12
